vi "Main.vi"() -> ()   [LabVIEW 2015]
doc: "This template is for the Queued Message Handler design pattern.\n\nThe Event Handling Loop generates messages based on user interface actions.\n\nThe Message Handling Loop processes messages generated by the Event Handling Loop, or by other messages. The messages are string values, so new messages can be added easily to the Message Cases case structure in the Message Handling Loop. Each message cluster can also provide an optional value for Message Data, which is a variant that can be converted to whatever message-specific data is required."
uses:
  controls/UI Data.ctl
  support/Message Queue/Message Queue.lvlib
  <vilib>/Utility/error.llb/Error Cluster From Error Code.vi
  support/User Event - Stop/User Event - Stop.lvlib
  support/Message Queue/Enqueue Message (Single).vi
  <vilib>/ErrorRing/Error Ring.xnode
  <vilib>/Utility/miscctls.llb/LVPointTypeDef.ctl
  controls/Case Status.ctl
  <vilib>/addons/database/NI_Database_API.lvlib
  <userlib>/Adding Configurations and lists/Get and Set Data.lvlib
  <userlib>/origin_lib_main/DB_Interface/DB Interface.lvlib
  <userlib>/origin_lib_main/DB_Interface/DB Operations Enum.ctl
  controls/Operation type.ctl
  controls/Type.ctl
  controls/Back to Business.ctl
  controls/Declined.ctl
  controls/Program.ctl
  controls/Date to query in report.ctl
  controls/Amount in query for report.ctl
  controls/Query for report Cluster.ctl
  <vilib>/Utility/NIReport.llb/NI_report.lvclass
  <vilib>/addons/_office/NI_ReportGenerationToolkit.lvlib
  controls/Date.ctl
  controls/Add New Case.ctl
  <vilib>/addons/_office/excel.llb/Excel Easy Table (str).vi
  <vilib>/Utility/config.llb/NI_LVConfig.lvlib
  controls/Global.vi
  <vilib>/Utility/config.llb/Write Key (Path).vi
  <vilib>/Utility/config.llb/Read Key (Path).vi
  <vilib>/addons/database/Connection.llb/DB Tools Open Connec (String).vi
  <userlib>/_OpenG.lib/array/array.llb/Remove Duplicates from 1D Array (String)__ogtk.vi
  controls/Update Case.ctl
panel:
  out "error out 11":errorcluster
  out "error out 10":errorcluster
  out "Array 3":string[][](array[string])
  out "Array 2":string[][](array[string])
  out "error out 9":errorcluster
  out "Array":string[][](array[string])
  out "error out 8":errorcluster
  out "error out 7":errorcluster
  out "error out 6":errorcluster
  in  "TAT RISK":bool
  out "data Out 2":variant[][](array[variant])
  out "data 2":string[][](array[string])
  out "DB Cols Names 2":string[](array[string])
  out "error out 5":errorcluster
  out "error out":errorcluster
  out "DB Cols Names":string[](array[string])
  out "data":string[][](array[string])
  out "data Out":variant[][](array[variant])
  out "error out 4":errorcluster
  out "String":string
  out "error out 3":errorcluster
  out "error out 2":errorcluster
  in  "Exit":bool
  in  "Home Button":bool
  out "Display <Replace Me>":string
  in  "Tab Control":T1(tab)
  in  "Add New Case":bool
  in  "Existing Case":bool
  in  "Report":bool
  in  "Save Button":bool
  in  "Attachement":path
  in  "New Case":T2 {"Business Replay date" format="%<%d/%m/%Y>T"; "Next Review date" format="%<%d/%m/%Y>T"; "Stamped date" format="%<%d/%m/%Y>T"; "CAD submission date" format="%<%d/%m/%Y>T"; "decline date" format="%<%d/%m/%Y>T"; "CAM date" format="%<%d/%m/%Y>T"; "Pending risk visit date" format="%<%d/%m/%Y>T"; "Back to business 3" format="%<%d/%m/%Y>T"; "Back to business 2" format="%<%d/%m/%Y>T"; "Back to business 1" format="%<%d/%m/%Y>T"; "3rd login Date" format="%<%d/%m/%Y>T"; "2nd login Date" format="%<%d/%m/%Y>T"; "1st Login Date" format="%<%d/%m/%Y>T"}
  in  "Delete Case":bool
  in  "Query by serial":bool
  in  "Case Serial":string
  in  "Query by customer name":bool
  in  "Customer Name":string(combo)
  in  "Customer Number":string
  in  "Query by customer number":bool
  in  "Update existing Case":T9={"Customer Number"="", "UW"="", "UWTH"="", "Customer Name"="", "Program"="", "Amount"="", "CCRM"="", "CCRTH"="", "Type"="", "Case status"="Under Review", "1st Login Date"=timestamp(0 s since 1904-01-01), "2nd login Date"=timestamp(0 s since 1904-01-01), "3rd login Date"=timestamp(0 s since 1904-01-01), "Back to business 1"=timestamp(0 s since 1904-01-01), "Back to business 2"=timestamp(0 s since 1904-01-01), "Back to business 3"=timestamp(0 s since 1904-01-01), "Pending risk visit date"=timestamp(0 s since 1904-01-01), "CAM date"=timestamp(0 s since 1904-01-01), "decline date"=timestamp(0 s since 1904-01-01), "CAD submission date"=timestamp(0 s since 1904-01-01), "Stamped date"=timestamp(0 s since 1904-01-01), "Next Review date"=timestamp(0 s since 1904-01-01), "Business Replay date"=timestamp(0 s since 1904-01-01), "Comment"="", "Declined"="", "Back to business"="", "serial"=""} {"Business Replay date" format="%<%d/%m/%Y>T"; "Next Review date" format="%<%d/%m/%Y>T"; "Stamped date" format="%<%d/%m/%Y>T"; "CAD submission date" format="%<%d/%m/%Y>T"; "decline date" format="%<%d/%m/%Y>T"; "CAM date" format="%<%d/%m/%Y>T"; "Pending risk visit date" format="%<%d/%m/%Y>T"; "Back to business 3" format="%<%d/%m/%Y>T"; "Back to business 2" format="%<%d/%m/%Y>T"; "Back to business 1" format="%<%d/%m/%Y>T"; "3rd login Date" format="%<%d/%m/%Y>T"; "2nd login Date" format="%<%d/%m/%Y>T"; "1st Login Date" format="%<%d/%m/%Y>T"}
  in  "attachement":string
  in  "Open attachement":bool
  out "Case Serial 2":string
  in  "Update":bool
  in  "Reset Button":bool
  in  "Report Tab":T10(tab)
  in  "Generic Report Tab":bool
  in  "Daily Report Tab":bool
  in  "review date before 90 days":bool
  in  "Reset Button 2":bool
  in  "Report Button":bool
  in  "Back":bool
  in  "Report Cluster":T11 {"Business Replay date"."From :" format="%<%d/%m/%y>T"; "Business Replay date"."To :" format="%<%d/%m/%y>T"; "Next Review date"."From :" format="%<%d/%m/%y>T"; "Next Review date"."To :" format="%<%d/%m/%y>T"; "Stamped date"."From :" format="%<%d/%m/%y>T"; "Stamped date"."To :" format="%<%d/%m/%y>T"; "CAD submission date"."From :" format="%<%d/%m/%y>T"; "CAD submission date"."To :" format="%<%d/%m/%y>T"; "decline date"."From :" format="%<%d/%m/%y>T"; "decline date"."To :" format="%<%d/%m/%y>T"; "CAM date"."From :" format="%<%d/%m/%y>T"; "CAM date"."To :" format="%<%d/%m/%y>T"; "Pending risk visit date"."From :" format="%<%d/%m/%y>T"; "Pending risk visit date"."To :" format="%<%d/%m/%y>T"; "Back to business 3"."From :" format="%<%d/%m/%y>T"; "Back to business 3"."To :" format="%<%d/%m/%y>T"; "Back to business 2"."From :" format="%<%d/%m/%y>T"; "Back to business 2"."To :" format="%<%d/%m/%y>T"; "Back to business 1"."From :" format="%<%d/%m/%y>T"; "Back to business 1"."To :" format="%<%d/%m/%y>T"; "3rd login Date"."From :" format="%<%d/%m/%y>T"; "3rd login Date"."To :" format="%<%d/%m/%y>T"; "2nd login Date"."From :" format="%<%d/%m/%y>T"; "2nd login Date"."To :" format="%<%d/%m/%y>T"; "1st Login Date"."From :" format="%<%d/%m/%y>T"; "1st Login Date"."To :" format="%<%d/%m/%y>T"}
  in  "Back":bool
  in  "Approved Date":T12 {"From :" format="%<%d/%m/%y>T"; "To :" format="%<%d/%m/%y>T"}
  in  "Report Button 3":bool
  in  "decline date":T12 {"From :" format="%<%d/%m/%y>T"; "To :" format="%<%d/%m/%y>T"}
  # "Underwriting Pipline Submission"
  # "Attachment:"
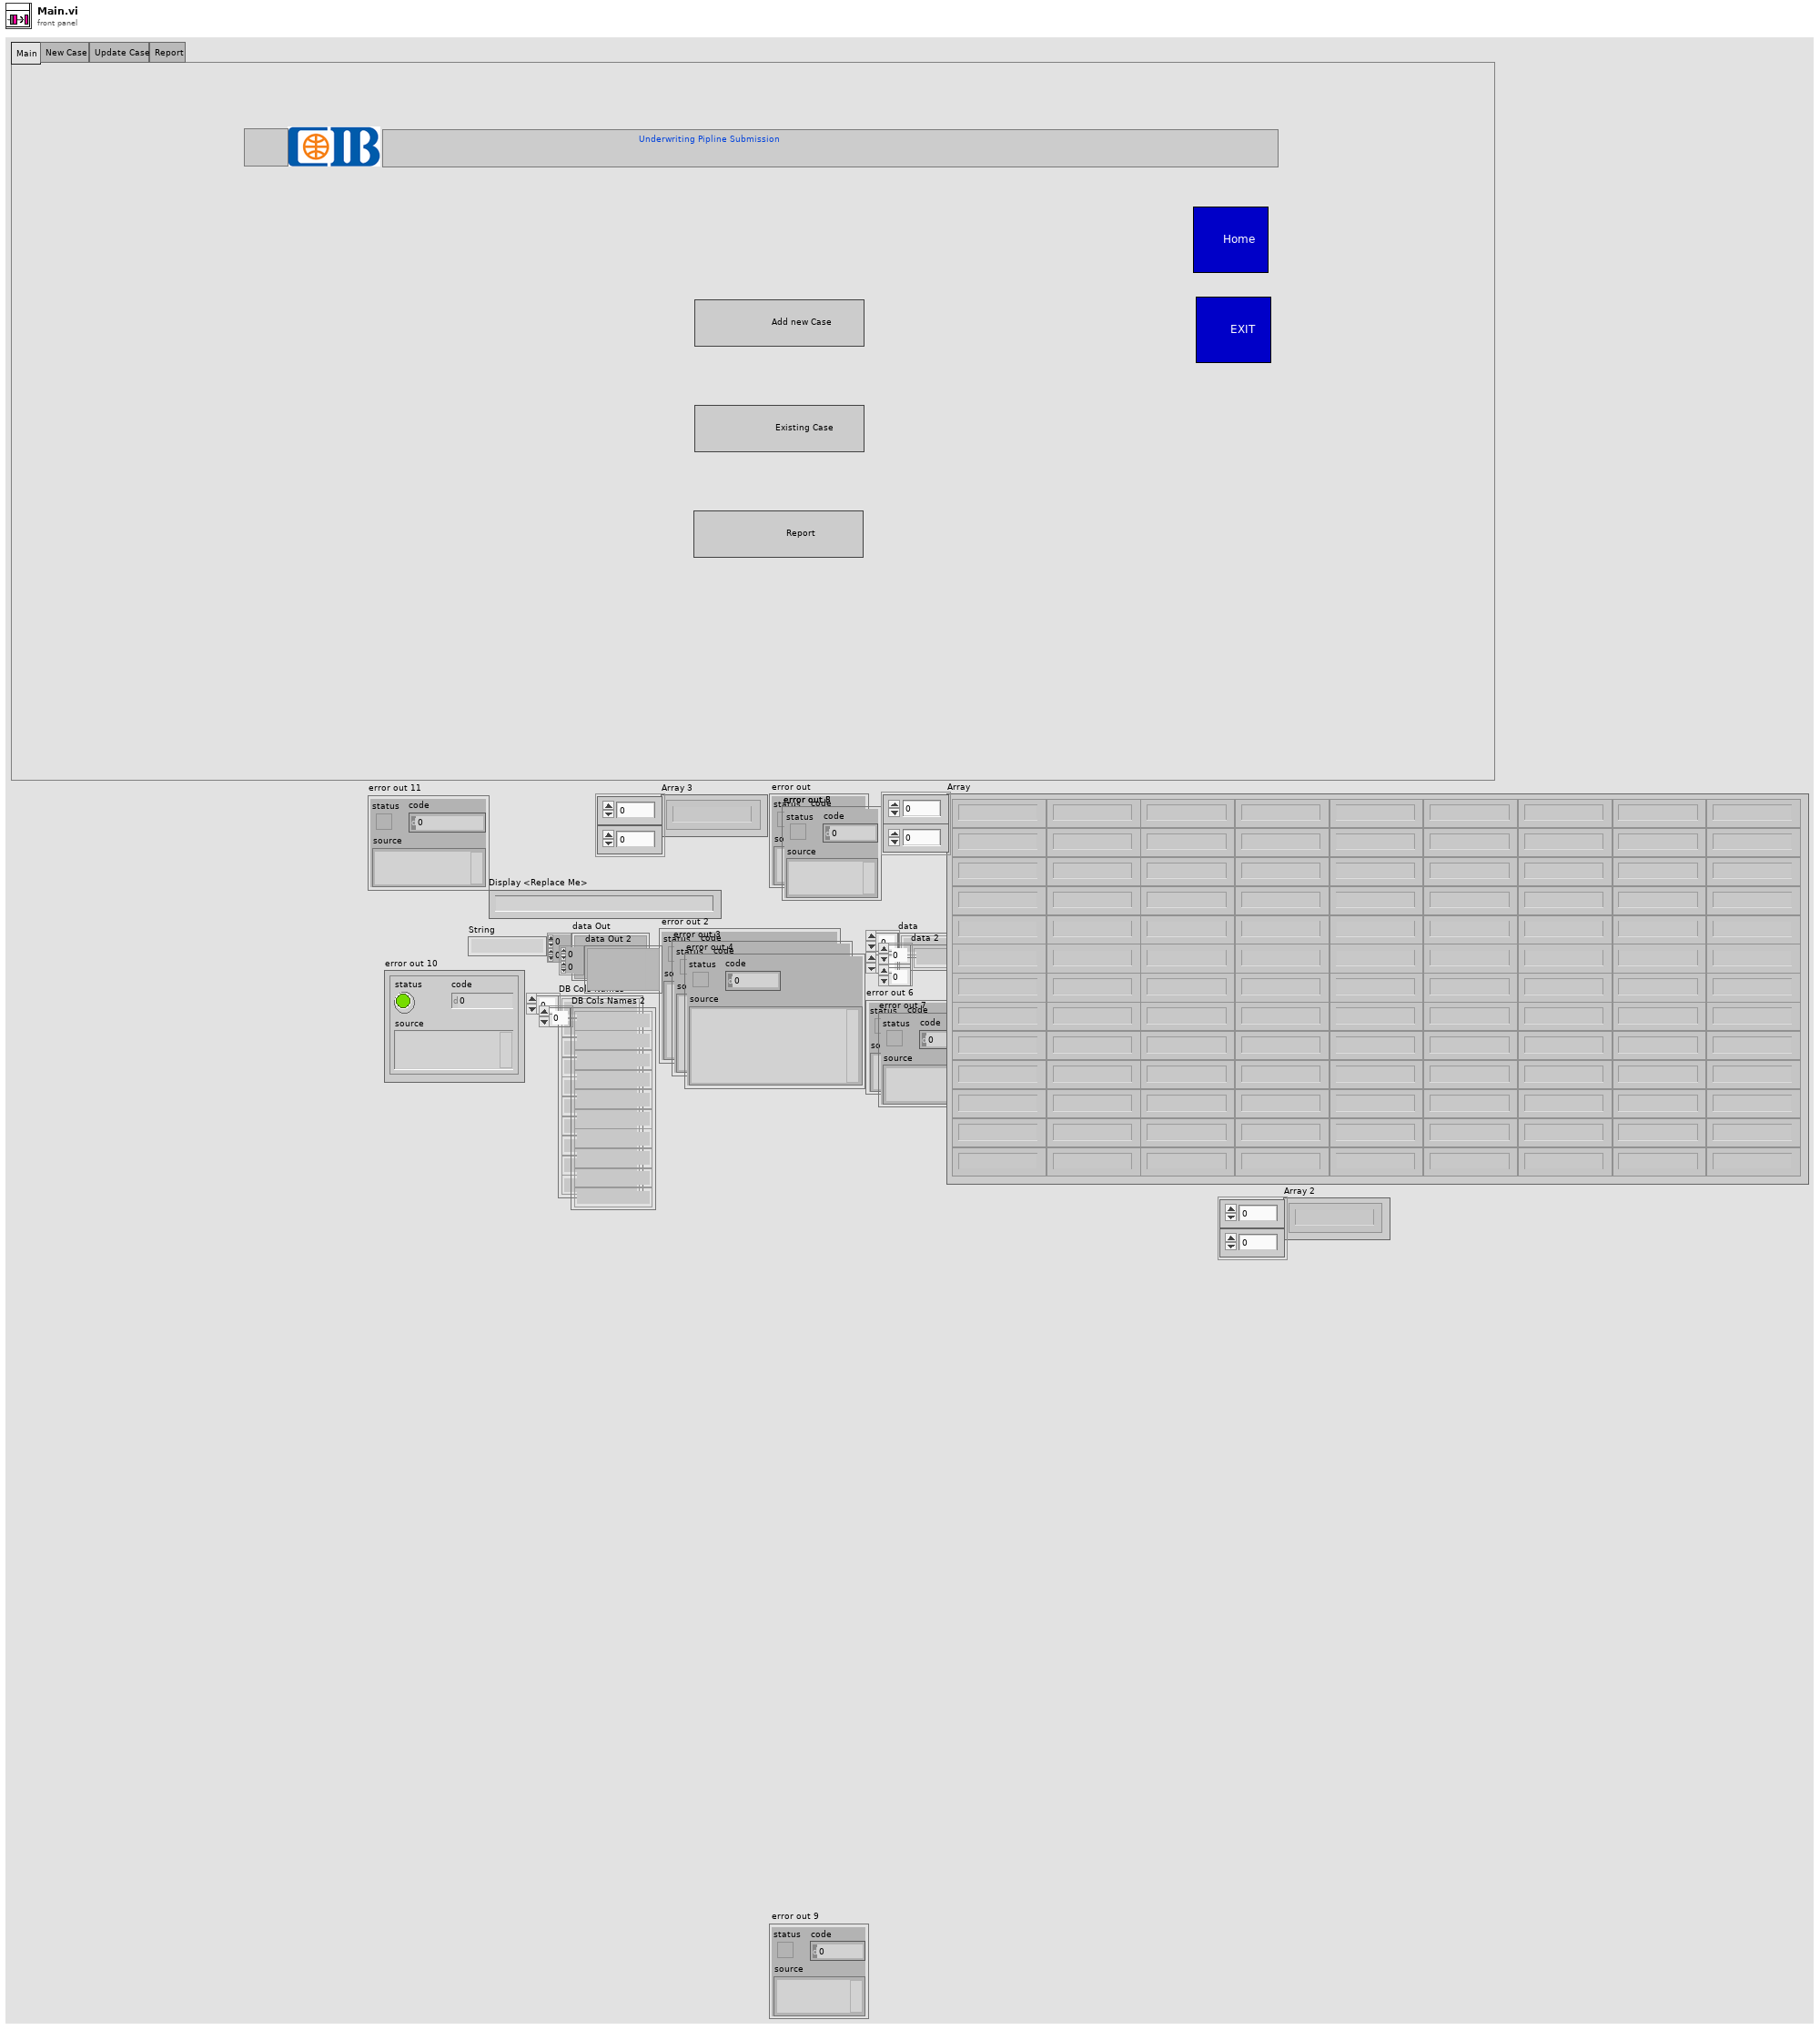
[diagram p1: front panel]
types:
  T1 = enum32{"Main", "New Case", "Update Case", "Report"}
  T2 = typedef "Add New Case.ctl" = cluster{"Customer Number":string, "UW":string, "UWTH":string, "Customer Name":string, "Program":T3, "Amount":string, "CCRM":string, "CCRTH":string, "Type":T4, "Case status":T5, "1st Login Date":T6, "2nd login Date":T6, "3rd login Date":T6, "Back to business 1":T6, "Back to business 2":T6, "Back to business 3":T6, "Pending risk visit date":T6, "CAM date":T6, "decline date":T6, "CAD submission date":T6, "Comment":string, "Stamped date":T6, "Next Review date":T6, "Declined":T7, "Back to business":T8, "serial":string, "Business Replay date":T6}
  T3 = typedef "Program.ctl" = string
  T4 = typedef "Type.ctl" = string
  T5 = typedef "Case Status.ctl" = string
  T6 = typedef "Date.ctl" = timestamp
  T7 = typedef "Declined.ctl" = string
  T8 = typedef "Back to Business.ctl" = string
  T9 = typedef "Update Case.ctl" = cluster{"Customer Number":string, "UW":string, "UWTH":string, "Customer Name":string, "Program":T3, "Amount":string, "CCRM":string, "CCRTH":string, "Type":T4, "Case status":T5, "1st Login Date":T6, "2nd login Date":T6, "3rd login Date":T6, "Back to business 1":T6, "Back to business 2":T6, "Back to business 3":T6, "Pending risk visit date":T6, "CAM date":T6, "decline date":T6, "CAD submission date":T6, "Stamped date":T6, "Next Review date":T6, "Business Replay date":T6, "Comment":string, "Declined":T7, "Back to business":T8, "serial":string}
  T10 = enum32{"Main Report", "Report 1", "Daily Report"}
  T11 = typedef "Query for report Cluster.ctl" = cluster{"UW":string, "UWTH":string, "CCRM":string, "CCRTH":string, "Type":T4, "Back to business":T8, "Declined":T7, "Program":T3, "Case status":T5, "1st Login Date":T12, "2nd login Date":T12, "3rd login Date":T12, "Business Replay date":T12, "Back to business 1":T12, "Back to business 2":T12, "Back to business 3":T12, "Next Review date":T12, "CAD submission date":T12, "CAM date":T12, "Pending risk visit date":T12, "decline date":T12, "Stamped date":T12, "Amount":T13, "Customer Number":string, "Customer Name":string, "Comment":string, "serial":string}
  T12 = typedef "Date to query in report.ctl" = cluster{"To :":timestamp, "From : ":timestamp}
  T13 = typedef "Amount in query for report.ctl" = cluster{"Amount":string, "Comparison":string}
  T14 = typedef "UI Data.ctl" = cluster{"Boolean <Replace Me>":bool, "String <Replace Me>":string, "Numeric <Replace Me>":dbl, "Do Something Ref":refnum<vi>, "Do Something Else Ref":refnum<vi>, "Data Display Ref":refnum<vi>, "Exit Button Ref":refnum<vi>}
  T15 = typedef "Message Queue.lvlib/All Message Queues.ctl" = cluster{"UI":refnum<queue>}
  T16 = typedef "LVDateTimeRec.ctl" = cluster{"fractional second":dbl, "second":i32, "minute":i32, "hour":i32, "day of month":i32, "month":i32, "year":i32, "day of week":i32, "day of year":i32, "DST":i32}
  T17 = enum8{"Enabled", "Disabled", "Disabled and Grayed Out"}
  T18 = typedef "LVPointTypeDef.ctl" = cluster{"Horizontal":i16, "Vertical":i16}
  T19 = typedef "Operation type.ctl" = enum16{"Add", "Query", "Update"}
  T20 = typedef "DB Interface.lvlib/DB Operations Enum.ctl" = enum16{"Select", "Update", "Insert", "Delete", "Fetch SQL Query", "Execute SQL Query", "Drop Table", "List Tables"}
  T21 = enum16{"Standard Report", "HTML", "Word", "Excel"}
  T22 = enum16{"maximized", "minimized", "normal", "no change"}
  T23 = typedef "NI_LVConfig.lvlib/Config Data RefNum.ctl" = refnum<k1>
  T24 = typedef "NI_Database_API.lvlib/Conn ObjectReference.ctl" = refnum<k1>
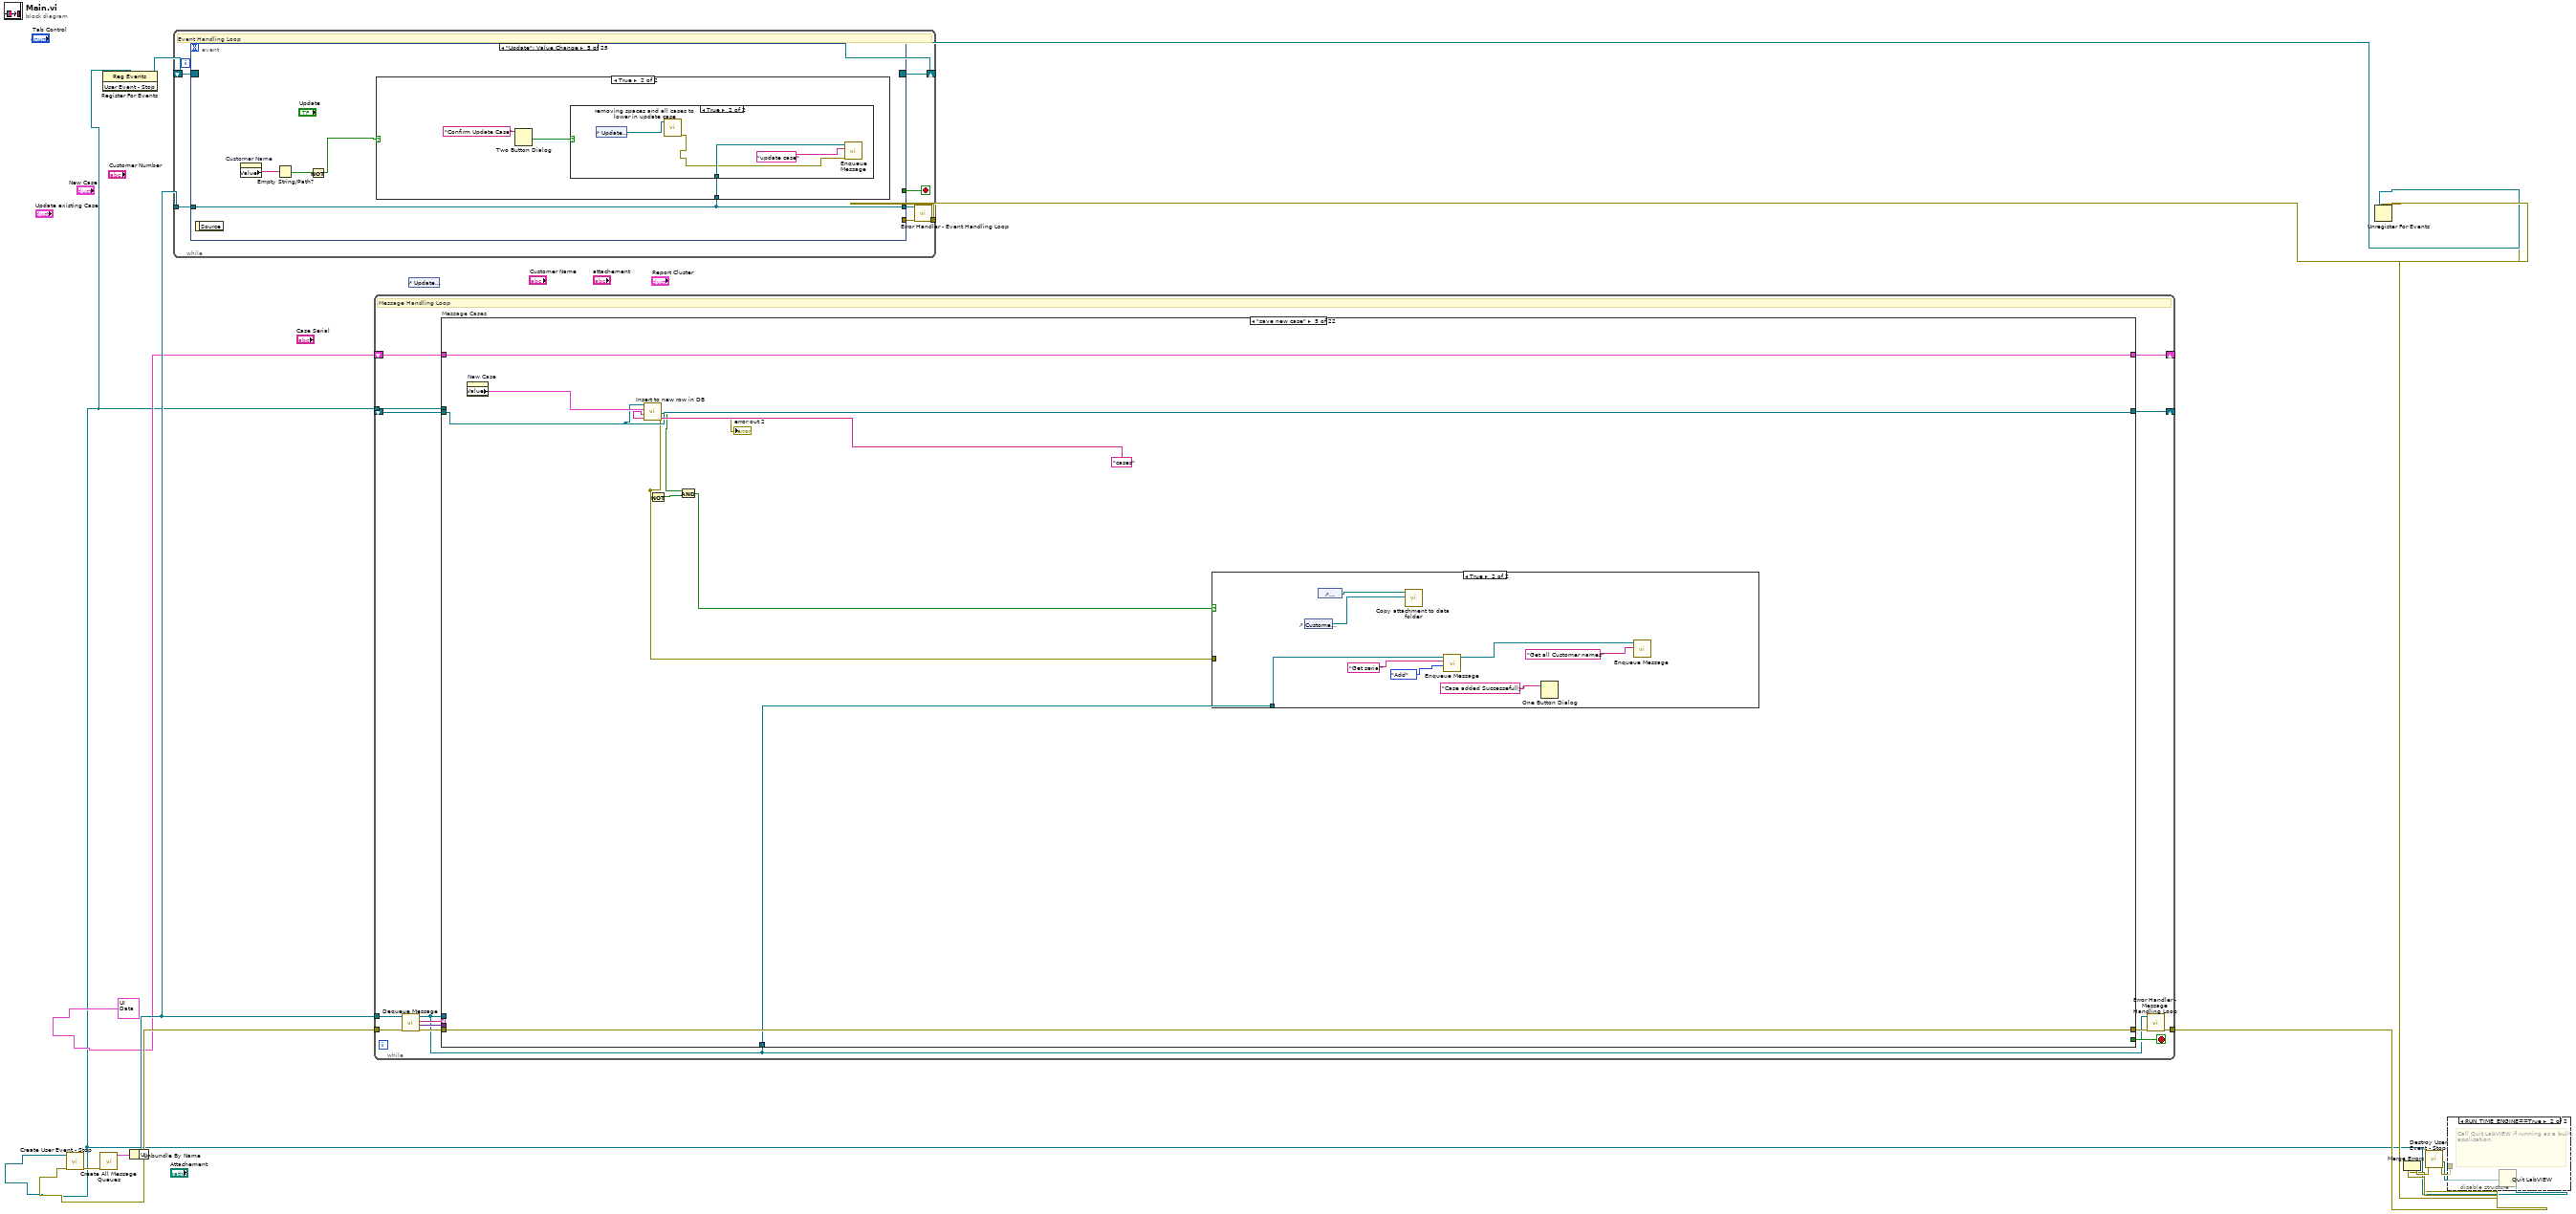
[diagram p0: block diagram]
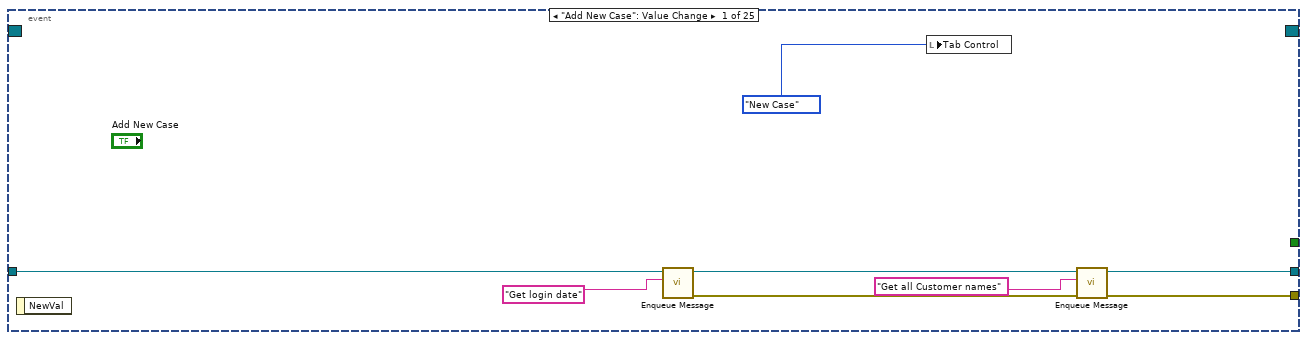
[diagram p3: hidden frame]
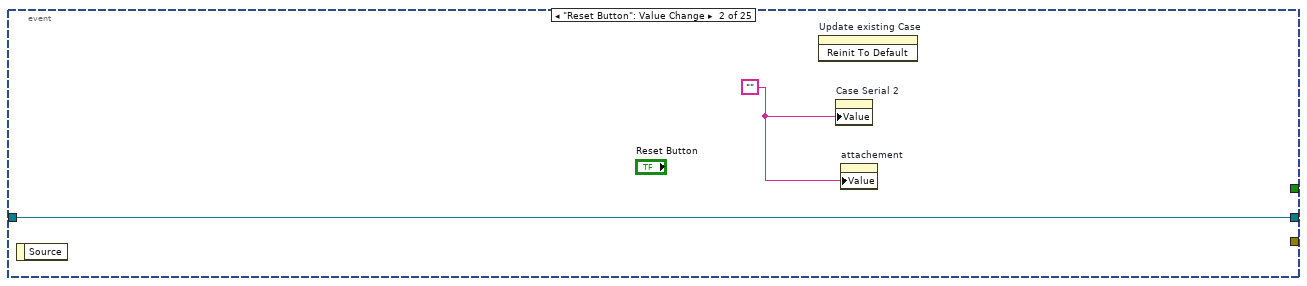
[diagram p4: hidden frame]
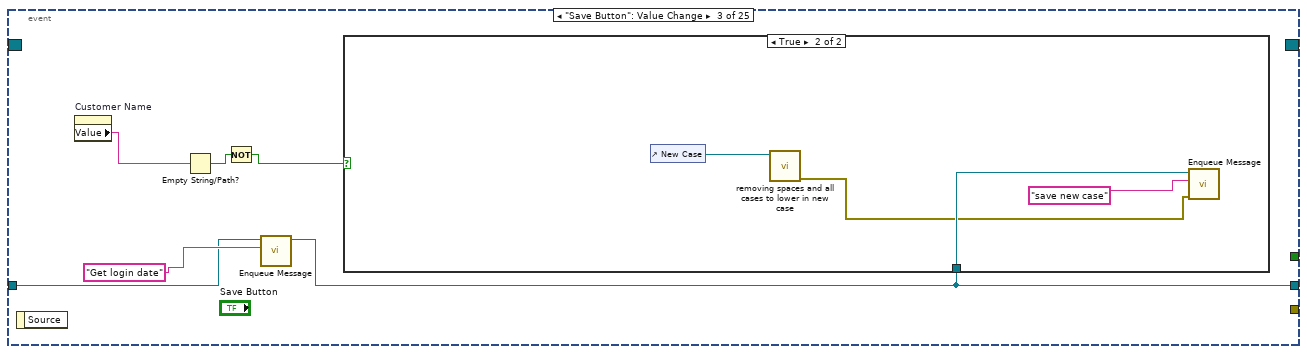
[diagram p5: hidden frame]
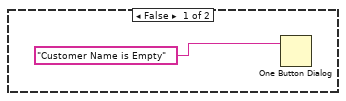
[diagram p6: hidden frame]
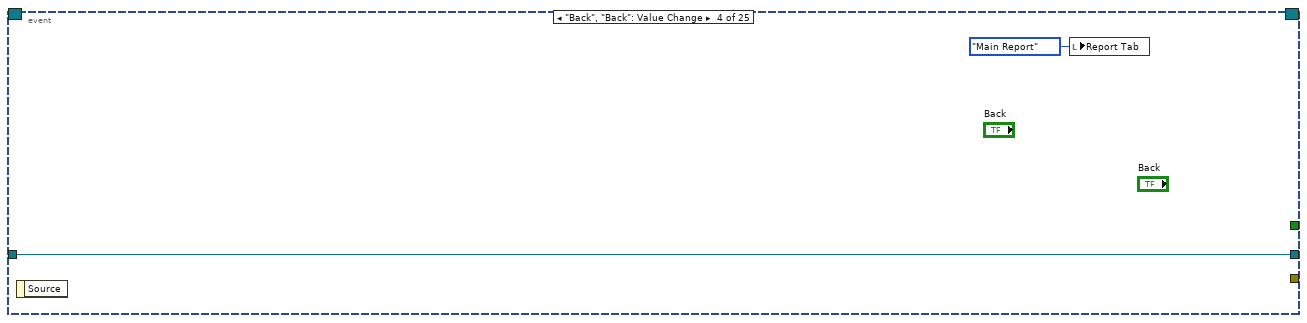
[diagram p7: hidden frame]
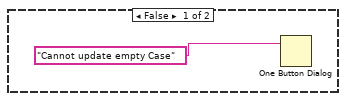
[diagram p8: hidden frame]
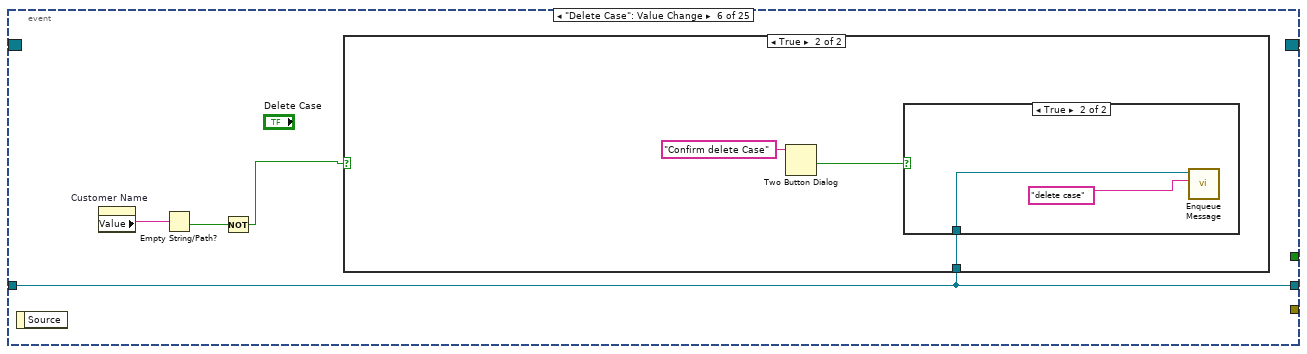
[diagram p10: hidden frame]
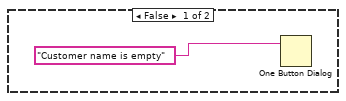
[diagram p11: hidden frame]
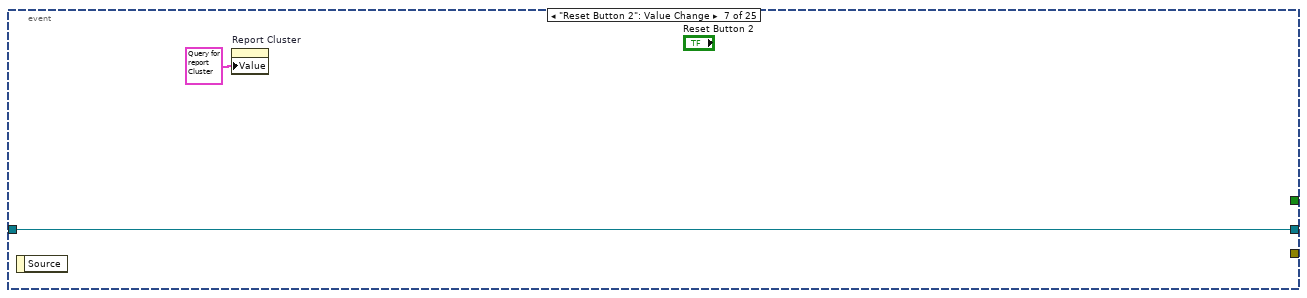
[diagram p13: hidden frame]
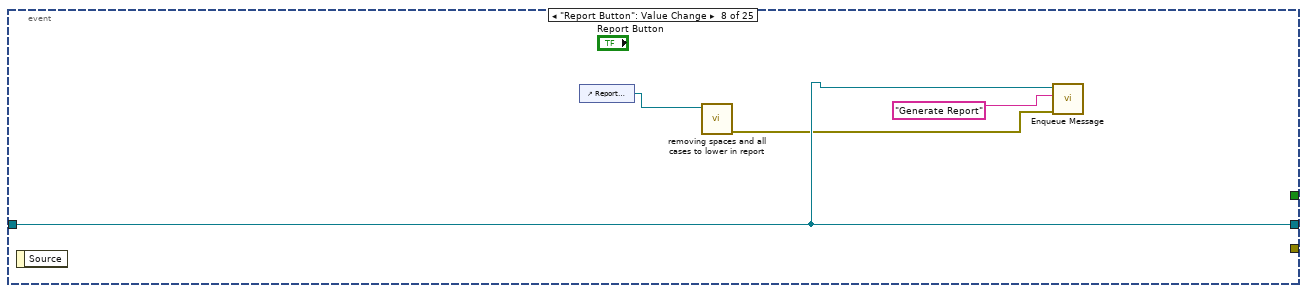
[diagram p14: hidden frame]
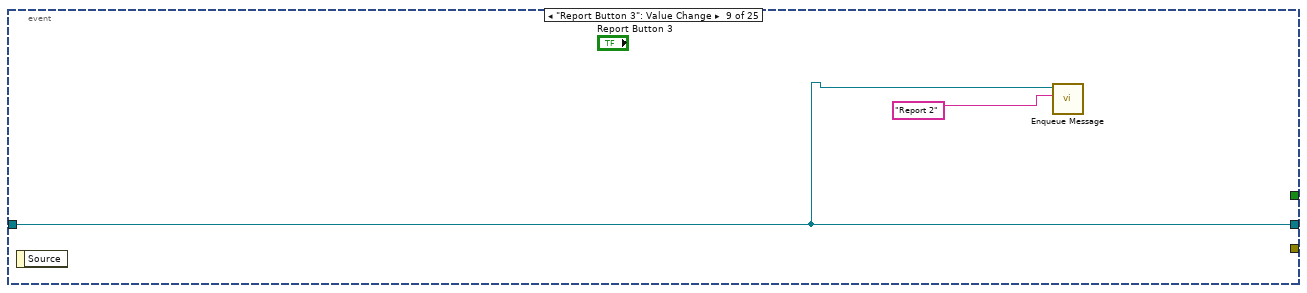
[diagram p15: hidden frame]
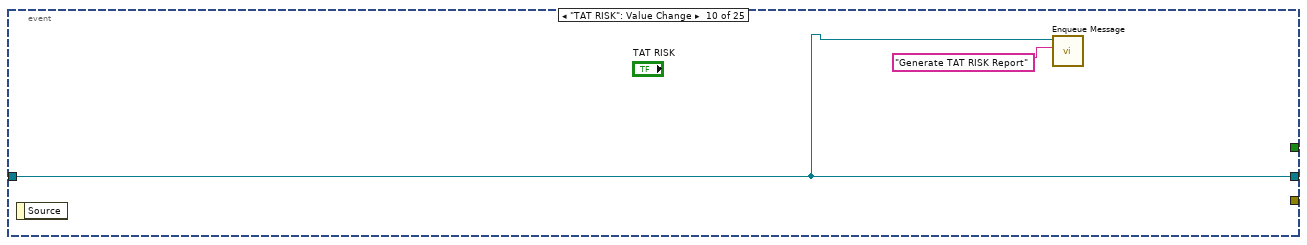
[diagram p16: hidden frame]
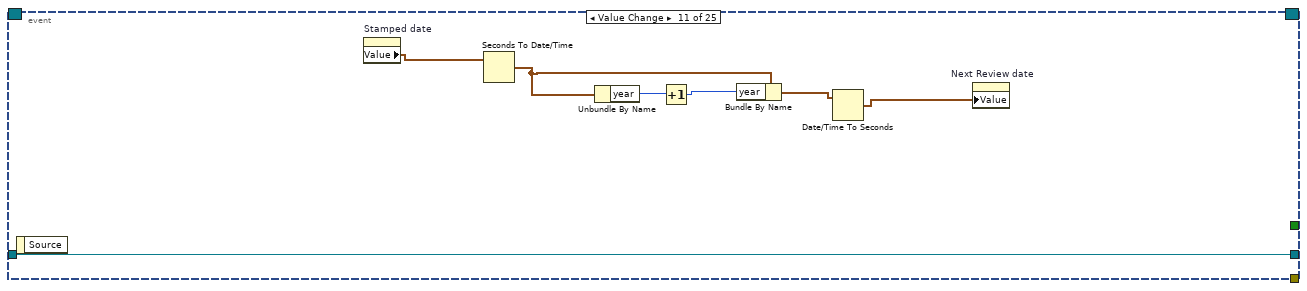
[diagram p17: hidden frame]
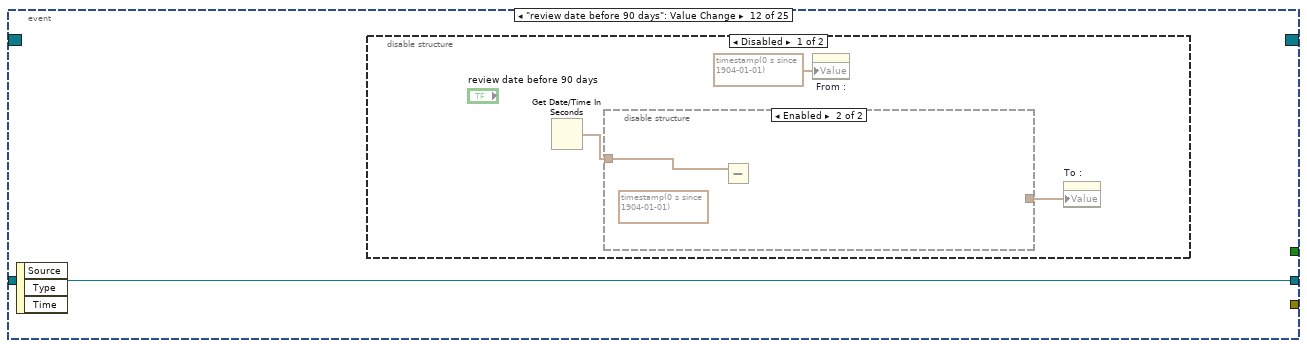
[diagram p18: hidden frame]
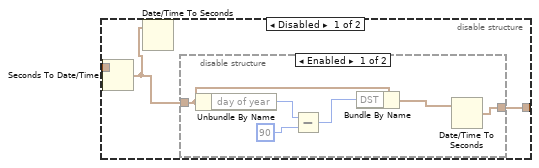
[diagram p19: hidden frame]
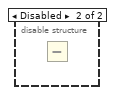
[diagram p20: hidden frame]
diagram:
  n1 = call "Create User Event - Stop.vi"() -> ("error out"=w9:errorcluster, "User Event - Stop"=w1:refnum<user-event>)  [unwired: 10 in]
  n2 = call "Create All Message Queues.vi"("error in (no error)"=w9) -> ("error out"=w13:errorcluster, "Message Queues out"=w12:T15)  [unwired: 9 in]
  n3 = register-events(w1) -> (reference out=w2:refnum<event-registration>)  [unwired: 2 in, 1 out]
  n4 = Unbundle By Name(w12) -> ("UI"=w10:refnum<queue>)
  n5 = while {
    tunnel: w10 -> [w20]
    shift-right: [w18] -> w6
    shift-left: w2 -> [w19]
    tunnel: [w14] -> w3
    stop <- w16 stop-if-true
    # "Event Handling Loop"
    n6 = event shown="[4] \"Update\": Value Change" {
      selector: w19 -> [_ _ _ _ _ _ _ _ _ _ _ _ _ _ _ _ _ _ _ _ _ _ _ _ _]
      dyn-events: [_ _ _ _ _ _ _ _ _ _ _ _ _ _ _ _ _ _ _ _ _ _ _ _ _] -> w18
      timeout: _ -> [_ _ _ _ _ _ _ _ _ _ _ _ _ _ _ _ _ _ _ _ _ _ _ _ _]
      tunnel: [_ _ _ _ _ _ _ _ _ _ _ _ _ _ _ _ _ _ _ _ _ _ _ _ TRUE ("Discard?")] -> w16
      tunnel: w20 -> [w28 w30 w32 w43 w47 w59 w67 w70 w72 w74 w82 w83 w111 w118 w121 w125 w132 w138 w141 w144 w146 w151 w153 w158 w161]
      tunnel: [w21 _ _ _ _ _ _ _ _ _ _ _ _ _ _ _ w129 w135 _ _ _ w150 _ w157 _] -> w17
      tunnel: [w23 w30 w31 w43 w47 w59 w67 w70 w72 w74 w82 w83 w111 w118 w121 w125 w131 w137 w141 w144 w146 w149 w153 w156 w161] -> w15
      event "Add New Case": Value Change {
        n7 = event-data() -> ()  [unwired: 1 in, 1 out]
        n8 = call-poly "Enqueue Message.vi"("Message"="Get login date", "Message Queue"=w28) -> ("error out"=w22:errorcluster, "dup Message Queue"=w24:refnum<queue>)  [unwired: 8 in]
        n9 = local write "Tab Control"(T1."New Case" ("Tab Control")) -> ()
        n10 = call-poly "Enqueue Message.vi"("error in (no error)"=w22, "Message"="Get all Customer names", "Message Queue"=w24) -> ("error out"=w21:errorcluster, "dup Message Queue"=w23:refnum<queue>)  [unwired: 7 in]
      }
      event "Reset Button": Value Change {
        w29 = ""
        n11 = event-data() -> ()  [unwired: 1 in, 1 out]
        n12 = invoke on="Update existing Case" class="Clust (strict)" method="Reinit To Default"() -> ()  [unwired: 3 in, 3 out]
        n13 = property on="Case Serial 2" class="Str"("Value"=w29) -> ()  [unwired: 2 in, 2 out]
        n14 = property on="attachement" class="Str"("Value"=w29) -> ()  [unwired: 2 in, 2 out]
      }
      event "Save Button": Value Change {
        n15 = event-data() -> ()  [unwired: 1 in, 1 out]
        n16 = property on="Customer Name" class="Str"() -> ("Value"=w36:string)  [unwired: 2 in, 2 out]
        n17 = Empty String/Path?(string/path=w36) -> (empty?=w35:bool)
        n18 = Not(x=w35) -> (.not. x?=w34:bool)
        n19 = call-poly "Enqueue Message.vi"("Message"="Get login date", "Message Queue"=w32) -> ("dup Message Queue"=w31:refnum<queue>)  [unwired: 8 in, 1 out]
        n20 = case shown="True" w34 {
          tunnel: w31 -> [_ w40]
          frame False {
            n21 = One Button Dialog(message="Customer Name is Empty") -> ()  [unwired: 1 in, 1 out]
          }
          frame True {
            n22 = control-ref of="New Case"() -> (w39:refnum<vi>)
            n23 = call "removing spaces and all cases to lower in new case.vi"("New Case"=w39) -> ("Error Out"=w38:errorcluster)  [unwired: 10 in]
            n24 = call-poly "Enqueue Message.vi"("error in (no error)"=w38, "Message"="save new case", "Message Queue"=w40) -> ()  [unwired: 7 in, 2 out]
          }
        }
      }
      event "Back", "Back": Value Change {
        n25 = event-data() -> ()  [unwired: 1 in, 1 out]
        n26 = local write "Report Tab"(T10."Main Report" ("Report Tab")) -> ()
      }
      event "Update": Value Change {
        n27 = event-data() -> ()  [unwired: 1 in, 1 out]
        n28 = property on="Customer Name" class="Str"() -> ("Value"=w46:string)  [unwired: 2 in, 2 out]
        n29 = Empty String/Path?(string/path=w46) -> (empty?=w45:bool)
        n30 = Not(x=w45) -> (.not. x?=w44:bool)
        n31 = case shown="True" w44 {
          tunnel: w47 -> [_ w51]
          frame False {
            n32 = One Button Dialog(message="Cannot update empty Case") -> ()  [unwired: 1 in, 1 out]
          }
          frame True {
            n33 = Two Button Dialog(message="Confirm Update Case") -> (T button?=w50:bool)  [unwired: 2 in]
            n34 = case shown="True" w50 {
              tunnel: w51 -> [_ w54]
              frame False {
              }
              frame True {
                n35 = control-ref of="Update existing Case"() -> (w53:refnum<vi>)
                n36 = call "removing spaces and all cases to lower in update case.vi"("Update existing Case"=w53) -> ("Error Out"=w52:errorcluster)  [unwired: 10 in]
                n37 = call-poly "Enqueue Message.vi"("error in (no error)"=w52, "Message"="update case", "Message Queue"=w54) -> ()  [unwired: 7 in, 2 out]
              }
            }
          }
        }
      }
      event "Delete Case": Value Change {
        n38 = event-data() -> ()  [unwired: 1 in, 1 out]
        n39 = property on="Customer Name" class="Str"() -> ("Value"=w58:string)  [unwired: 2 in, 2 out]
        n40 = Empty String/Path?(string/path=w58) -> (empty?=w57:bool)
        n41 = Not(x=w57) -> (.not. x?=w56:bool)
        n42 = case shown="True" w56 {
          tunnel: w59 -> [_ w63]
          frame False {
            n43 = One Button Dialog(message="Customer name is empty") -> ()  [unwired: 1 in, 1 out]
          }
          frame True {
            n44 = Two Button Dialog(message="Confirm delete Case") -> (T button?=w62:bool)  [unwired: 2 in]
            n45 = case shown="True" w62 {
              tunnel: w63 -> [_ w64]
              frame False {
              }
              frame True {
                n46 = call-poly "Enqueue Message.vi"("Message"="delete case", "Message Queue"=w64) -> ()  [unwired: 8 in, 2 out]
              }
            }
          }
        }
      }
      event "Reset Button 2": Value Change {
        n47 = event-data() -> ()  [unwired: 1 in, 1 out]
        n48 = property on="Report Cluster" class="Clust (strict)"("Value"=T11 {"UW"="", "UWTH"="", "CCRM"="", "CCRTH"="", "Type"="", "Back to business"="", "Declined"="", "Program"="", "Case status"="", "1st Login Date"={"To :"=timestamp(0 s since 1904-01-01), "From : "=timestamp(0 s since 1904-01-01)}, "2nd login Date"={"To :"=timestamp(0 s since 1904-01-01), "From : "=timestamp(0 s since 1904-01-01)}, "3rd login Date"={"To :"=timestamp(0 s since 1904-01-01), "From : "=timestamp(0 s since 1904-01-01)}, "Business Replay date"={"To :"=timestamp(0 s since 1904-01-01), "From : "=timestamp(0 s since 1904-01-01)}, "Back to business 1"={"To :"=timestamp(0 s since 1904-01-01), "From : "=timestamp(0 s since 1904-01-01)}, "Back to business 2"={"To :"=timestamp(0 s since 1904-01-01), "From : "=timestamp(0 s since 1904-01-01)}, "Back to business 3"={"To :"=timestamp(0 s since 1904-01-01), "From : "=timestamp(0 s since 1904-01-01)}, "Next Review date"={"To :"=timestamp(0 s since 1904-01-01), "From : "=timestamp(0 s since 1904-01-01)}, "CAD submission date"={"To :"=timestamp(0 s since 1904-01-01), "From : "=timestamp(0 s since 1904-01-01)}, "CAM date"={"To :"=timestamp(0 s since 1904-01-01), "From : "=timestamp(0 s since 1904-01-01)}, "Pending risk visit date"={"To :"=timestamp(0 s since 1904-01-01), "From : "=timestamp(0 s since 1904-01-01)}, "decline date"={"To :"=timestamp(0 s since 1904-01-01), "From : "=timestamp(0 s since 1904-01-01)}, "Stamped date"={"To :"=timestamp(0 s since 1904-01-01), "From : "=timestamp(0 s since 1904-01-01)}, "Amount"={"Amount"="", "Comparison"=""}, "Customer Number"="", "Customer Name"="", "Comment"="", "serial"=""} ("Update existing Case 2")) -> ()  [unwired: 2 in, 2 out]
      }
      event "Report Button": Value Change {
        n49 = event-data() -> ()  [unwired: 1 in, 1 out]
        n50 = control-ref of="Report Cluster"() -> (w69:refnum<vi>)
        n51 = call "removing spaces and all cases to lower in report.vi"("Report Cluster"=w69) -> ("Error Out"=w68:errorcluster)  [unwired: 10 in]
        n52 = call-poly "Enqueue Message.vi"("error in (no error)"=w68, "Message"="Generate Report", "Message Queue"=w70) -> ()  [unwired: 7 in, 2 out]
      }
      event "Report Button 3": Value Change {
        n53 = event-data() -> ()  [unwired: 1 in, 1 out]
        n54 = call-poly "Enqueue Message.vi"("Message"="Report 2", "Message Queue"=w72) -> ()  [unwired: 8 in, 2 out]
      }
      event "TAT RISK": Value Change {
        n55 = event-data() -> ()  [unwired: 1 in, 1 out]
        n56 = call-poly "Enqueue Message.vi"("Message"="Generate TAT RISK Report", "Message Queue"=w74) -> ()  [unwired: 8 in, 2 out]
      }
      event Value Change {
        n57 = event-data() -> ()  [unwired: 1 in, 1 out]
        n58 = property on="Stamped date" class="AbsTime (strict)"() -> ("Value"=w76:T6)  [unwired: 2 in, 2 out]
        n59 = Seconds To Date/Time(time stamp (now)=w76) -> (date time rec=w80:T16)  [unwired: 1 in]
        n60 = Unbundle By Name(w80) -> ("year"=w81:i32)
        n61 = Increment(x=w81) -> (x+1=w79:i32)
        n62 = Bundle By Name(cluster=w80, "year"=w79) -> (w78:T16)
        n63 = Date/Time To Seconds(2:w78) -> (0:w77:timestamp)  [unwired: 1 in]
        n64 = property on="Next Review date" class="AbsTime (strict)"("Value"=w77) -> ()  [unwired: 2 in, 2 out]
      }
      event "review date before 90 days": Value Change {
        n65 = event-data() -> ()  [unwired: 1 in, 3 out]
        n66 = disable-structure shown="Disabled" {
          frame Disabled {
            n67 = Get Date/Time In Seconds() -> (seconds since 1Jan1904=w85:timestamp)
            n68 = disable-structure shown="Enabled" {
              disable-tunnel: w85 -> [w89 w96]
              disable-tunnel: [w88 _] -> w84
              frame Disabled {
                n69 = Seconds To Date/Time(time stamp (now)=w89) -> (date time rec=w87:T16)  [unwired: 1 in]
                n70 = Date/Time To Seconds(2:w87) -> ()  [unwired: 1 in, 1 out]
                n71 = disable-structure shown="Enabled" {
                  disable-tunnel: w87 -> [w95 _]
                  disable-tunnel: [w90 _] -> w88
                  frame Enabled {
                    n72 = Unbundle By Name(w95) -> ("day of year"=w94:i32)
                    n73 = Subtract(x=w94, y=90) -> (x-y=w92:i32)
                    n74 = Bundle By Name(cluster=w95, "DST"=w92) -> (w91:T16)
                    n75 = Date/Time To Seconds(2:w91) -> (0:w90:timestamp)  [unwired: 1 in]
                  }
                  frame Disabled {
                    n76 = Subtract() -> ()  [unwired: 2 in, 1 out]
                  }
                }
              }
              frame Enabled {
                (unwired) timestamp(0 s since 1904-01-01) ("seconds since 1Jan1904")
                n77 = Subtract(x=w96) -> ()  [unwired: 1 in, 1 out]
              }
            }
            n78 = property on="From :" class="AbsTime (strict)"("Value"=timestamp(0 s since 1904-01-01)) -> ()  [unwired: 2 in, 2 out]
            n79 = property on="To :" class="AbsTime (strict)"("Value"=w84) -> ()  [unwired: 2 in, 2 out]
          }
          frame Enabled {
          }
        }
      }
      event "Open attachement": Value Change {
        n80 = event-data() -> ()  [unwired: 1 in, 1 out]
        n81 = global read "Global.vi" "attachment path"() -> (w97:path)
        n82 = property on="attachement" class="Str"() -> ("Value"=w102:string)  [unwired: 2 in, 2 out]
        n83 = call <vilib>:"Is Path and Not Empty.vi"("path"=w97) -> ("Is Path and Not Empty?"=w98:bool)  [unwired: 4 in]
        n84 = property on="Customer Name" class="Str"() -> ("Value"=w100:string)  [unwired: 2 in, 2 out]
        n85 = case shown="True" w98 {
          tunnel: [w114 w115] -> w99
          tunnel: w97 -> [_ w115]
          frame False {
            n86 = call <vilib>:"Application Directory.vi"() -> ("Application Directory"=w113:path)
            n87 = Build Path(base path=w113, name or relative path="data\\attachment\\") -> (appended path=w114:path)
          }
          frame True {
          }
        }
        n88 = Concatenate Strings(w100, "\\", w102) -> (w110:string)
        n89 = Build Path(base path=w99, name or relative path=w110) -> (appended path=w103:path)
        n90 = Path To String(path=w103) -> (string=w108:string)
        n91 = Concatenate Strings("cmd  /c \"", w108, "\"") -> (w106:string)
        n92 = call <vilib>:"System Exec.vi"("run minimized? (F)"=TRUE, "wait until completion? (T)"=FALSE, "command line"=w106) -> ()  [unwired: 5 in, 4 out]
      }
      event "Query by customer number": Value Change {
        n93 = event-data() -> ()  [unwired: 1 in, 1 out]
        n94 = property on="Customer Number" class="Str"() -> ("Value"=w117:string)  [unwired: 2 in, 2 out]
        n95 = Empty String/Path?(string/path=w117) -> (empty?=w116:bool)
        n96 = case shown="False" w116 {
          tunnel: w118 -> [w119 _]
          frame False {
            n97 = call-poly "Enqueue Message.vi"("Message"="Query by customer number", "Message Queue"=w119) -> ()  [unwired: 8 in, 2 out]
          }
          frame True {
          }
        }
      }
      event "Query by serial": Value Change {
        n98 = event-data() -> ()  [unwired: 1 in, 1 out]
        n99 = call-poly "Enqueue Message.vi"("Message"="Query by serial", "Message Queue"=w121) -> ()  [unwired: 8 in, 2 out]
      }
      event "Query by customer name": Value Change {
        n100 = event-data() -> ()  [unwired: 1 in, 1 out]
        n101 = property on="Customer Name" class="CmbBox"() -> ("Value"=w124:string)  [unwired: 2 in, 2 out]
        n102 = Empty String/Path?(string/path=w124) -> (empty?=w123:bool)
        n103 = case shown="False" w123 {
          tunnel: w125 -> [w126 _]
          frame False {
            n104 = call-poly "Enqueue Message.vi"("Message"="Query by customer name", "Message Queue"=w126) -> ()  [unwired: 8 in, 2 out]
          }
          frame True {
          }
        }
      }
      event "Existing Case": Value Change {
        n105 = event-data() -> ()  [unwired: 1 in, 1 out]
        n106 = call-poly "Enqueue Message.vi"("Message"="Get all Customer names", "Message Queue"=w132) -> ("error out"=w129:errorcluster, "dup Message Queue"=w131:refnum<queue>)  [unwired: 8 in]
        n107 = local write "Tab Control"(T1."Update Case" ("Tab Control")) -> ()
      }
      event "Report": Value Change {
        n108 = event-data() -> ()  [unwired: 1 in, 1 out]
        n109 = call-poly "Enqueue Message.vi"("Message"="Get all Customer names", "Message Queue"=w138) -> ("error out"=w135:errorcluster, "dup Message Queue"=w137:refnum<queue>)  [unwired: 8 in]
        n110 = local write "Report Tab"(T10."Main Report" ("Report Tab")) -> ()
        n111 = local write "Tab Control"(T1."Report" ("Tab Control")) -> ()
      }
      event "Generic Report Tab": Value Change {
        n112 = event-data() -> ()  [unwired: 1 in, 1 out]
        n113 = local write "Report Tab"(T10."Report 1" ("Report Tab")) -> ()
        n114 = local write "Tab Control"(T1."Report" ("Tab Control")) -> ()
      }
      event "Daily Report Tab": Value Change {
        n115 = event-data() -> ()  [unwired: 1 in, 1 out]
        n116 = local write "Report Tab"(T10."Daily Report" ("Report Tab")) -> ()
        n117 = local write "Tab Control"(T1."Report" ("Tab Control")) -> ()
      }
      event "Home Button": Value Change {
        n118 = event-data() -> ()  [unwired: 1 in, 1 out]
        n119 = local write "Tab Control"(T1."Main" ("Tab Control")) -> ()
      }
      event Panel Close? {
        # "Send the 'Confirm Quit' message if the user closes the panel of the VI. Discard the event so the 'Confirm Quit' message has a chance to run."
        n120 = event-data() -> ()  [unwired: 1 in, 1 out]
        n121 = call-poly "Enqueue Message.vi"("Priority Message? (F)"=TRUE, "Message"="Confirm Quit", "Message Queue"=w151) -> ("error out"=w150:errorcluster, "dup Message Queue"=w149:refnum<queue>)  [unwired: 7 in]
        n122 = event-data("Discard?"=TRUE) -> ()  [unwired: 1 in, 1 out]
      }
      event Application Instance Close {
        # "#CodeRecommended - When a project closes, all VIs within that project are aborted and leave memory. However, any code placed in this event frame is guaranteed to run to completion, so add any cleanup code that absolutely must happen here."
        n123 = event-data() -> ()  [unwired: 1 in, 1 out]
      }
      event "Exit": Value Change {
        n124 = event-data() -> ()  [unwired: 1 in, 1 out]
        n125 = call-poly "Enqueue Message.vi"("Priority Message? (F)"=TRUE, "Message"="Exit", "Message Queue"=w158) -> ("error out"=w157:errorcluster, "dup Message Queue"=w156:refnum<queue>)  [unwired: 7 in]
      }
      event User Event {
        # "The Message Handling Loop processed an \"Exit\" message, which fired this event to stop the Event Handling Loop."
        n126 = event-data() -> ()  [unwired: 1 in, 1 out]
        n127 = local write "Display <Replace Me>"("\"Exit\" button pressed" ("VI Stopped")) -> ()
      }
    }
    n128 = call "Error Handler - Event Handling Loop.vi"("error in (no error)"=w17, "Message Queue"=w15) -> ("dup error in"=w14:errorcluster)  [unwired: 8 in, 1 out]
  }
  n129 = while {
    tunnel: w10 -> [w167]
    shift-right: [w174] -> _
    shift-left: T14 {"Boolean <Replace Me>"=FALSE, "String <Replace Me>"="", "Numeric <Replace Me>"=0.0, "Do Something Ref"=refnum, "Do Something Else Ref"=refnum, "Data Display Ref"=refnum, "Exit Button Ref"=refnum} ("Data Cluster") -> [w175]
    tunnel: w1 -> [w172]
    tunnel: w13 -> [w171]
    tunnel: [w166] -> w11
    shift-right: [w164] -> _
    shift-left: _ -> [w163]
    stop <- w173 stop-if-true
    # "Message Handling Loop"
    n130 = call "Dequeue Message.vi"("error in (no error)"=w171, "Message Queue"=w167) -> ("error out"=w170:errorcluster, "Message Data"=w168:variant, "Message"=w169:string, "dup Message Queue"=w162:refnum<queue>)  [unwired: 6 in]
    n131 = case "Message Cases" shown="\"save new case\"" w169 {
      selector: w169 -> [_ _ _ _ _ _ _ _ _ _ _ _ _ _ _ _ _ _ _ _ _ w646]
      tunnel: w162 -> [w184 _ _ _ _ _ _ w319 _ w351 w368 _ _ _ _ w600 _ _ w624 _ w644 _]
      tunnel: w170 -> [w191 w210 w231 w252 w272 w298 w313 w326 w344 w358 w373 w394 w406 w464 w569 w602 w610 w620 w628 w632 w637 _]
      tunnel: [w192 w210 w232 w253 w272 w298 w313 w326 w344 w358 w373 w394 w406 w464 w569 w603 w611 w614 w626 w630 w640 w647] -> w165
      tunnel: w175 -> [w190 w209 w233 w254 w271 w297 w312 w325 w343 w357 w372 w393 w405 w463 w568 w604 w612 w619 w627 w631 w643 w648]
      tunnel: [w189 w209 w233 w254 w271 w297 w312 w325 w343 w357 w372 w393 w405 w463 w568 w604 w612 w619 w627 w631 w643 w648] -> w174
      tunnel: [_ _ _ _ _ _ _ _ _ _ _ _ _ _ _ _ _ _ _ _ TRUE _] -> w173
      tunnel: w168 -> [_ _ _ w241 _ _ _ _ _ _ _ _ _ _ _ _ w609 w618 _ _ w634 _]
      tunnel: w172 -> [_ _ _ _ _ _ _ _ _ _ _ _ _ _ _ _ _ _ _ _ w639 _]
      tunnel: [w176 w207 w230 w251 w268 w295 w311 w323 w342 w355 w370 w391 w397 w441 w565 w597 w605 w613 w621 w629 w633 w645] -> w164
      tunnel: w163 -> [w176 _ w230 w251 w268 w295 w311 w323 w342 w355 w370 w391 w397 w441 w565 w597 w605 w613 w621 w629 w633 w645]
      tunnel: w162 -> [_ _ _ _ w263 _ _ _ _ _ _ _ _ _ _ _ _ _ _ _ _ _]
      frame "Initialize" {
        # "Initialize - All initialization work should take place in this message, since other loops can potentially enqueue messages that execute immediately after this one."
        n132 = control-ref of="Exit"() -> (w182:refnum<vi>)
        n133 = control-ref of="Add New Case"() -> (w188:refnum<vi>)
        n134 = control-ref of="Existing Case"() -> (w187:refnum<vi>)
        n135 = control-ref of="Display <Replace Me>"() -> (w186:refnum<vi>)
        n136 = control-ref of="Pane"() -> (w181:refnum<vi>)
        n137 = property on="Case status" class="CmbBox (strict)"("Value"=T5 "Under Review", "DisabledEnum"=T17."Disabled and Grayed Out" ("Disabled")) -> ()  [unwired: 2 in, 2 out]
        n138 = Bundle By Name(cluster=w190, "Do Something Ref"=w188, "Do Something Else Ref"=w187, "Data Display Ref"=w186, "Exit Button Ref"=w182, "String <Replace Me>"="Initial Message" ("Initial Message")) -> (w189:T14)
        n139 = property class="Pane"(reference=w181, "Origin"=T18 {"Horizontal"=0, "Vertical"=0}) -> ()  [unwired: 1 in, 2 out]
        n140 = control-ref of="This VI"() -> (w179:refnum<vi>)
        n141 = invoke class="VI" method="Default Vals.Reinit All"(reference=w179) -> ()  [unwired: 2 in, 3 out]
        n142 = call-poly "Enqueue Message.vi"("error in (no error)"=w191, "Message"="Init DB", "Message Queue"=w184) -> ("error out"=w192:errorcluster)  [unwired: 7 in, 1 out]
      }
      frame "Init DB" {
        # "open DB"
        # "Install DB file"
        # "create ODBC"
        n143 = call <vilib>:"Application Directory.vi"() -> ("Application Directory"=w200:path)
        n144 = Build Path(base path=w200, name or relative path="data\\config.ini") -> (appended path=w197:path)
        n145 = call <vilib>:"Open Config Data.vi"("configuration file path"=w197) -> ("file created?"=w199:bool, "refnum"=w198:T23)  [unwired: 8 in, 1 out]
        n146 = case shown="True" w199 {
          tunnel: w198 -> [_ w218]
          tunnel: [_ w214] -> w195
          frame False {
          }
          frame True {
            n147 = call "DialogUsingEvents 1.vi"() -> ("Attachment path"=w212:path)  [unwired: 10 in, 1 out]
            n148 = call <vilib>:"Is Path and Not Empty.vi"("path"=w212) -> ("Is Path and Not Empty?"=w213:bool)  [unwired: 4 in]
            n149 = case shown="False" w213 {
              tunnel: [w221 w222] -> w211
              tunnel: w212 -> [_ w222]
              frame False {
                n150 = call <vilib>:"Application Directory.vi"() -> ("Application Directory"=w220:path)
                n151 = Build Path(base path=w220, name or relative path="data\\attachment\\") -> (appended path=w221:path)
              }
              frame True {
              }
            }
            n152 = call-poly <vilib>:"Write Key.vi"("section"="attachment", "value"=w211, "key"="path", "refnum"=w218) -> ("refnum out"=w215:T23)  [unwired: 5 in, 2 out]
            n153 = call <vilib>:"Close Config Data.vi"("refnum"=w215) -> ("error out"=w214:errorcluster)  [unwired: 9 in, 1 out]
          }
        }
        n154 = call-poly <vilib>:"DB Tools Open Connection.vi"("connection information"="Underwriting Pipline Submission") -> ("connection reference"=w207:T24)  [unwired: 7 in, 1 out]
        n155 = call <vilib>:"Open Config Data.vi"("error in (no error)"=w195, "configuration file path"=w197) -> ("refnum"=w196:T23)  [unwired: 7 in, 2 out]
        n156 = call <vilib>:"Application Directory.vi"() -> ("Application Directory"=w204:path)
        n157 = Build Path(base path=w204, name or relative path="data\\attachment\\") -> (appended path=w202:path)
        n158 = call "SQL Commands.vi"("connection reference"=w207) -> ()  [unwired: 9 in, 2 out]
        n159 = call-poly <vilib>:"Read Key.vi"("section"="attachment", "default value"=w202, "key"="path", "refnum"=w196) -> ("value"=w193:path, "refnum out"=w194:T23)  [unwired: 4 in, 2 out]
        n160 = global write "Global.vi" "attachment path"(w193) -> ()
        n161 = call <vilib>:"Close Config Data.vi"("refnum"=w194) -> ()  [unwired: 9 in, 2 out]
      }
      frame "Get login date" {
        # "Something - Replace this message with functionality for your own application."
        n162 = Get Date/Time In Seconds() -> (seconds since 1Jan1904=w229:timestamp)
        n163 = Seconds To Date/Time(time stamp (now)=w229) -> (date time rec=w224:T16)  [unwired: 1 in]
        n164 = Unbundle By Name(w224) -> ("hour"=w228:i32)
        n165 = Greater Or Equal?(x=w228, y=12) -> (x >= y?=w225:bool)
        n166 = case shown="True" w225 {
          tunnel: w224 -> [w234 w238]
          tunnel: [w234 w235] -> w223
          frame False {
          }
          frame True {
            n167 = Unbundle By Name(w238) -> ("day of month"=w237:i32)
            n168 = Increment(x=w237) -> (x+1=w236:i32)
            n169 = Bundle By Name(cluster=w238, "day of month"=w236) -> (w235:T16)
          }
        }
        n170 = Date/Time To Seconds(2:w223) -> (0:w226:timestamp)  [unwired: 1 in]
        n171 = property on="1st Login Date" class="AbsTime (strict)"("Value"=w226) -> ()  [unwired: 2 in, 2 out]
        n172 = Merge Errors(w231) -> (w232:errorcluster)
      }
      frame "Get serial" {
        # "Something - Replace this message with functionality for your own application."
        n173 = Variant To Data(type=Operation_type."Add", Variant=w241) -> (data=w239:T19)  [unwired: 1 in, 1 out]
        n174 = case shown="\"Add\"" w239 {
          tunnel: [w255 w256] -> w244
          frame "Add" {
            n175 = property on="Customer Name" class="Str"() -> ("Value"=w255:string)  [unwired: 2 in, 2 out]
          }
          frame "Query", Default {
            n176 = property on="Customer Name" class="Str"() -> ("Value"=w256:string)  [unwired: 2 in, 2 out]
          }
        }
        n177 = Format Into String(format string="where Customer_Name = '%s'", w244) -> (resulting string=w245:string)  [unwired: 2 in, 1 out]
        n178 = call <userlib>:"DB Interface.vi"("DB Ref In"=w251, "Operation"=DB_Operations_Enum."Select", "condition"=w245, "DB Table"="cases", "DB columns"=string[] ["id"]) -> ("data Out"=w247:variant[][])  [unwired: 7 in, 3 out]
        n179 = call <userlib>:"Variant to String.vi"("Var"=w247) -> ("String"=w242:string)  [unwired: 9 in, 1 out]
        "String" <- w242
        n180 = Merge Errors(w252) -> (w253:errorcluster)
        n181 = case shown="\"Update\"" w239 {
          tunnel: "Case serial : " -> [w260 _ _]
          tunnel: w242 -> [w258 w262 _]
          frame "Add", Default {
            n182 = Concatenate Strings(w260, w258) -> (w259:string)
            n183 = One Button Dialog(message=w259) -> (true=w257:bool)  [unwired: 1 in]
            n184 = case shown="True" w257 {
              frame False {
              }
              frame True {
                n185 = invoke on="Attachement" class="Path" method="Reinit To Default"() -> ()  [unwired: 3 in, 3 out]
                n186 = property on="New Case" class="Clust (strict)"("Value"=T2 {"Customer Number"="", "UW"="", "UWTH"="", "Customer Name"="", "Program"="", "Amount"="", "CCRM"="", "CCRTH"="", "Type"="", "Case status"="Under Review", "1st Login Date"=timestamp(3720200378.523235 s since 1904-01-01), "2nd login Date"=timestamp(0 s since 1904-01-01), "3rd login Date"=timestamp(0 s since 1904-01-01), "Back to business 1"=timestamp(0 s since 1904-01-01), "Back to business 2"=timestamp(0 s since 1904-01-01), "Back to business 3"=timestamp(0 s since 1904-01-01), "Pending risk visit date"=timestamp(0 s since 1904-01-01), "CAM date"=timestamp(0 s since 1904-01-01), "decline date"=timestamp(0 s since 1904-01-01), "CAD submission date"=timestamp(0 s since 1904-01-01), "Comment"="", "Stamped date"=timestamp(0 s since 1904-01-01), "Next Review date"=timestamp(0 s since 1904-01-01), "Declined"="", "Back to business"="", "serial"="", "Business Replay date"=timestamp(0 s since 1904-01-01)} ("New Case")) -> ()  [unwired: 2 in, 2 out]
              }
            }
          }
          frame "Query" {
            n187 = property on="Case Serial 2" class="Str"("Value"=w262) -> ()  [unwired: 2 in, 2 out]
          }
          frame "Update" {
          }
        }
      }
      frame "save new case" {
        n188 = property on="New Case" class="Clust (strict)"() -> ("Value"=w270:T2)  [unwired: 2 in, 2 out]
        n189 = call <userlib>:"Insert to new row in DB.vi"("connection reference"=w268, "Input Cluster"=w270, "table"="cases") -> ("Sucess ?"=w267:bool, "error out"=w264:errorcluster)  [unwired: 5 in, 1 out]
        "error out 2" <- w264
        n190 = Not(x=w264) -> (.not. x?=w266:bool)
        n191 = And(x=w267, y=w266) -> (x .and. y?=w265:bool)
        n192 = case shown="True" w265 {
          tunnel: w264 -> [w277 _]
          tunnel: w263 -> [_ w284]
          frame False {
            w274 = "Duplicate entry"
            n193 = Unbundle By Name(w277) -> ("source"=w276:string)
            n194 = Match Pattern(string=w276, regular expression=w274) -> (match substring=w275:string)  [unwired: 1 in, 3 out]
            n195 = Equal?(x=w275, y=w274) -> (x = y?=w273:bool)
            n196 = case shown="True" w273 {
              frame False {
              }
              frame True {
                n197 = One Button Dialog(message="Customer name must be unique") -> ()  [unwired: 1 in, 1 out]
              }
            }
            n198 = One Button Dialog(message="Error Inserting New Case") -> ()  [unwired: 1 in, 1 out]
          }
          frame True {
            n199 = control-ref of="Customer Name"() -> (w282:refnum<vi>)
            n200 = control-ref of="Attachement"() -> (w286:refnum<vi>)
            n201 = call "Copy attachment to data folder.vi"("Str Refnum"=w282, "Path in"=w286) -> ()  [unwired: 9 in, 1 out]
            n202 = call-poly "Enqueue Message.vi"("Message Data"=Operation_type."Add", "Message"="Get serial", "Message Queue"=w284) -> ("dup Message Queue"=w280:refnum<queue>)  [unwired: 7 in, 1 out]
            n203 = One Button Dialog(message="Case added Successefully") -> ()  [unwired: 1 in, 1 out]
            n204 = call-poly "Enqueue Message.vi"("Message"="Get all Customer names", "Message Queue"=w280) -> ()  [unwired: 8 in, 2 out]
          }
        }
      }
      frame "update case" {
        n205 = property on="Update existing Case" class="Clust (strict)"() -> ("Value"=w290:T9)  [unwired: 2 in, 2 out]
        n206 = property on="Case Serial 2" class="Str"() -> ("Value"=w288:string)  [unwired: 2 in, 2 out]
        n207 = Decimal String To Number(string=w288) -> (number=w289:i32)  [unwired: 2 in, 1 out]
        n208 = call <userlib>:"update data in DB.vi"("connection reference"=w295, "Input Cluster"=w290, "table"="cases", "Unique index"=w289) -> ("Sucess ?"=w294:bool, "error out"=w291:errorcluster)  [unwired: 4 in, 1 out]
        "error out 3" <- w291
        n209 = Not(x=w291) -> (.not. x?=w293:bool)
        n210 = And(x=w294, y=w293) -> (x .and. y?=w292:bool)
        n211 = case shown="True" w292 {
          tunnel: w291 -> [_ _]
          frame False {
            n212 = One Button Dialog(message="Error updating Case") -> ()  [unwired: 1 in, 1 out]
          }
          frame True {
            n213 = disable-structure shown="Enabled" {
              frame Enabled {
                w301 = ""
                n214 = property on="Case Serial 2" class="Str"("Value"=w301) -> ()  [unwired: 2 in, 2 out]
                n215 = property on="attachement" class="Str"("Value"=w301) -> ()  [unwired: 2 in, 2 out]
              }
              frame Disabled {
              }
            }
            n216 = disable-structure shown="Enabled" {
              frame Enabled {
                n217 = invoke on="Update existing Case" class="Clust (strict)" method="Reinit To Default"() -> ()  [unwired: 3 in, 3 out]
              }
              frame Disabled {
              }
            }
            n218 = One Button Dialog(message="Case updated Successefully") -> ()  [unwired: 1 in, 1 out]
          }
        }
      }
      frame "delete case" {
        n219 = property on="Customer Name" class="Str"() -> ("Value"=w302:string)  [unwired: 2 in, 2 out]
        n220 = Format Into String(format string="where Customer_Name ='%s'" ("condition"), w302) -> (resulting string=w303:string)  [unwired: 2 in, 1 out]
        n221 = call <userlib>:"DB Interface.vi"("DB Ref In"=w311, "Operation"=DB_Operations_Enum."Delete", "condition"=w303, "DB Table"="cases") -> ("Sucess ?"=w310:bool, "error out"=w307:errorcluster)  [unwired: 8 in, 2 out]
        "error out 4" <- w307
        n222 = Not(x=w307) -> (.not. x?=w309:bool)
        n223 = And(x=w310, y=w309) -> (x .and. y?=w308:bool)
        n224 = case shown="True" w308 {
          tunnel: w307 -> [_ _]
          frame False {
            n225 = One Button Dialog(message="Error deleting Case") -> ()  [unwired: 1 in, 1 out]
          }
          frame True {
            n226 = disable-structure shown="Enabled" {
              frame Enabled {
                w316 = ""
                n227 = property on="Case Serial 2" class="Str"("Value"=w316) -> ()  [unwired: 2 in, 2 out]
                n228 = property on="attachement" class="Str"("Value"=w316) -> ()  [unwired: 2 in, 2 out]
              }
              frame Disabled {
              }
            }
            n229 = disable-structure shown="Enabled" {
              frame Enabled {
                n230 = invoke on="Update existing Case" class="Clust (strict)" method="Reinit To Default"() -> ()  [unwired: 3 in, 3 out]
              }
              frame Disabled {
              }
            }
            n231 = One Button Dialog(message="Case deleted Successefully") -> ()  [unwired: 1 in, 1 out]
          }
        }
      }
      frame "Query by customer number" {
        n232 = property on="Customer Number" class="Str"() -> ("Value"=w321:string)  [unwired: 2 in, 2 out]
        n233 = control-ref of="Update existing Case"() -> (w318:refnum<vi>)
        n234 = call <userlib>:"Get Data by config name.vi"("config name"=w321, "index"=0, "variant"=w318, "table"="cases", "DB Ref In"=w323) -> ("Array"=w317:string[])  [unwired: 3 in, 3 out]
        n235 = Empty Array?(array=w317) -> (empty?=w320:bool)
        n236 = call "Get dates from DB.vi"("Update existing Case"=w318, "Array"=w317) -> ()  [unwired: 10 in]
        n237 = case shown="False" w320 {
          tunnel: w319 -> [w327 _]
          frame False {
            n238 = call-poly "Enqueue Message.vi"("Message"="Get attachement", "Message Queue"=w327) -> ()  [unwired: 8 in, 2 out]
            n239 = call-poly "Enqueue Message.vi"("Message Data"=Operation_type."Query", "Message"="Get serial", "Message Queue"=w327) -> ()  [unwired: 7 in, 2 out]
          }
          frame True {
            n240 = One Button Dialog(message="Case not found") -> ()  [unwired: 1 in, 1 out]
          }
        }
      }
      frame "Get attachement" {
        n241 = global read "Global.vi" "attachment path"() -> (w333:path)
        n242 = property on="Customer Name" class="Str"() -> ("Value"=w335:string)  [unwired: 2 in, 2 out]
        n243 = call <vilib>:"Is Path and Not Empty.vi"("path"=w333) -> ("Is Path and Not Empty?"=w334:bool)  [unwired: 4 in]
        n244 = case shown="False" w334 {
          tunnel: [w346 w348] -> w332
          tunnel: w333 -> [_ w348]
          frame False {
            n245 = call <vilib>:"Application Directory.vi"() -> ("Application Directory"=w347:path)
            n246 = Build Path(base path=w347, name or relative path="data\\attachment\\") -> (appended path=w346:path)
          }
          frame True {
          }
        }
        n247 = Concatenate Strings(w335, "\\") -> (w340:string)
        n248 = Build Path(base path=w332, name or relative path=w340) -> (appended path=w339:path)
        n249 = List Folder(path=w339) -> (filenames=w338:string[])  [unwired: 3 in, 3 out]
        n250 = Index Array(array=w338, index=0) -> (element=w336:string)
        n251 = property on="attachement" class="Str"("Value"=w336) -> ()  [unwired: 2 in, 2 out]
      }
      frame "Query by customer name" {
        n252 = control-ref of="Update existing Case"() -> (w349:refnum<vi>)
        n253 = property on="Customer Name" class="CmbBox"() -> ("Value"=w353:string)  [unwired: 2 in, 2 out]
        n254 = call <userlib>:"Get Data by config name.vi"("config name"=w353, "index"=3, "variant"=w349, "table"="cases", "DB Ref In"=w355) -> ("Array"=w350:string[])  [unwired: 3 in, 3 out]
        n255 = Empty Array?(array=w350) -> (empty?=w352:bool)
        n256 = call "Get dates from DB.vi"("Update existing Case"=w349, "Array"=w350) -> ()  [unwired: 10 in]
        n257 = case shown="False" w352 {
          tunnel: w351 -> [w359 _]
          frame False {
            n258 = call-poly "Enqueue Message.vi"("Message"="Get attachement", "Message Queue"=w359) -> ()  [unwired: 8 in, 2 out]
            n259 = call-poly "Enqueue Message.vi"("Message Data"=Operation_type."Query", "Message"="Get serial", "Message Queue"=w359) -> ()  [unwired: 7 in, 2 out]
          }
          frame True {
            n260 = One Button Dialog(message="Case not found") -> ()  [unwired: 1 in, 1 out]
          }
        }
      }
      frame "Query by serial" {
        n261 = control-ref of="Update existing Case"() -> (w366:refnum<vi>)
        n262 = property on="Case Serial" class="Str"() -> ("Value"=w365:string)  [unwired: 2 in, 2 out]
        n263 = Decimal String To Number(string=w365) -> (number=w364:i32)  [unwired: 2 in, 1 out]
        n264 = call <userlib>:"Get Config Data.vi"("Unique index"=w364, "variant"=w366, "table"="cases", "DB Ref"=w370) -> ("Array"=w367:string[])  [unwired: 5 in, 2 out]
        n265 = Empty Array?(array=w367) -> (empty?=w369:bool)
        n266 = call "Get dates from DB.vi"("Update existing Case"=w366, "Array"=w367) -> ()  [unwired: 10 in]
        n267 = case shown="True" w369 {
          tunnel: w368 -> [w374 _]
          frame False {
            n268 = call-poly "Enqueue Message.vi"("Message"="Get attachement", "Message Queue"=w374) -> ()  [unwired: 8 in, 2 out]
            n269 = call-poly "Enqueue Message.vi"("Message Data"=Operation_type."Query", "Message"="Get serial", "Message Queue"=w374) -> ()  [unwired: 7 in, 2 out]
          }
          frame True {
            n270 = One Button Dialog(message="Case not found") -> ()  [unwired: 1 in, 1 out]
          }
        }
      }
      frame "Get all Customer names" {
        n271 = call <userlib>:"DB Interface.vi"("DB Ref In"=w391, "Operation"=DB_Operations_Enum."Select", "DB Table"="cases", "DB columns"=string[] ["Customer_Name", "UW"]) -> ("data Out"=w388:variant[][])  [unwired: 8 in, 3 out]
        n272 = Variant To Data(type=string[][] [], Variant=w388) -> (data=w386:string[][])  [unwired: 1 in, 1 out]
        n273 = Index Array(array=w386, index (col) #1=0 ("disabled index (col)"), index (col) #2=1 ("index (col)")) -> (element #1=w384:string[], element #2=w380:string[])  [unwired: 2 in]
        n274 = call-poly <userlib>:"Remove Duplicates from 1D Array__ogtk.vi"("Input Array"=w380) -> ("Output Array"=w379:string[])  [unwired: 1 out]
        n275 = control-ref of="UW"() -> (w382:refnum<vi>)
        n276 = property class="CmbBox"(reference=w382, "Strings[]"=w379) -> (error out=→"error out 10":errorcluster)  [unwired: 1 in, 1 out]
        n277 = property on="Customer Name" class="CmbBox"("Strings[]"=w384) -> ()  [unwired: 2 in, 2 out]
        n278 = property on="UW" class="CmbBox"("Strings[]"=w379) -> ()  [unwired: 2 in, 2 out]
        n279 = property on="UW" class="CmbBox"("Strings[]"=w379) -> ()  [unwired: 2 in, 2 out]
      }
      frame "Generate Report" {
        w396 = "cases" ("DB Table")
        n280 = control-ref of="Report Cluster"() -> (w402:refnum<vi>)
        n281 = disable-structure shown="Enabled" {
          disable-tunnel: w402 -> [w433 _]
          disable-tunnel: [w432 _] -> w401
          frame Enabled {
            n282 = call "get condition.vi"("Report Cluster"=w433) -> ("Condition"=w432:string)  [unwired: 10 in]
          }
          frame Disabled {
          }
        }
        n283 = call <vilib>:"DB Tools List Columns.vi"("table"=w396, "connection reference"=w397) -> ("columns"=w395:string[])  [unwired: 2 in, 3 out]
        "DB Cols Names" <- w395
        n284 = call <userlib>:"DB Interface.vi"("DB Ref In"=w397, "Operation"=DB_Operations_Enum."Select", "condition"=w401, "DB Table"=w396) -> ("data Out"=w403:variant[][], "error out"=→"error out":errorcluster)  [unwired: 8 in, 2 out]
        "data Out" <- w403
        n285 = call <userlib>:"Variant to String 2D Array.vi"("data Out"=w403) -> ("data"=w399:string[][])  [unwired: 9 in, 1 out]
        "data" <- w399
        n286 = Empty Array?(array=w399) -> (empty?=w398:bool)
        n287 = case shown="False" w398 {
          tunnel: w395 -> [w420 _]
          tunnel: w401 -> [w412 _]
          tunnel: w399 -> [w410 _]
          frame False {
            n288 = for {
              tunnel: w410 -> [w422] mode=indexing
              tunnel: [w421] -> w411 mode=indexing
              n289 = for {
                tunnel: w422 -> [w424] mode=indexing
                tunnel: [w423] -> w421 mode=indexing
                n290 = Equal?(x=w424, y="1/1/1904" ("search string")) -> (x = y?=w428:bool)
                n291 = Equal?(x=w424, y="1/1/1600" ("search string")) -> (x = y?=w427:bool)
                n292 = Or(x=w428, y=w427) -> (x .or. y?=w426:bool)
                n293 = Select(t="NULL" ("search string"), s=w426, f=w424) -> (s? t:f=w423:string)
              }
            }
            n294 = call <vilib>:"New Report.vi"("report type"=T21."Excel") -> ("report out"=w408:refnum<class "NI_report.lvclass">)  [unwired: 13 in, 1 out]
            n295 = call <vilib>:"Application Directory.vi"() -> ("Application Directory"=w418:path)
            n296 = Build Path(base path=w418, name or relative path="data\\Reports\\") -> (appended path=w416:path)
            n297 = Concatenate Strings(w412, ".xls") -> (w415:string)
            n298 = Build Path(base path=w416, name or relative path=w415) -> (appended path=w413:path)
            n299 = call-poly <vilib>:"Excel Easy Table.vi"("report in"=w408, "text data"=w411, "column headers"=w420) -> ("report out"=w419:refnum<class "NI_report.lvclass">)  [unwired: 8 in, 4 out]
            n300 = call-dynamic "Save Report to File.vi"("report in"=w419, "report file path"=w413) -> ("error out"=→"error out 6":errorcluster)  [unwired: 12 in, 1 out]
          }
          frame True {
            n301 = One Button Dialog(message="No cases found with these conditions") -> ()  [unwired: 1 in, 1 out]
          }
        }
      }
      frame "Report 2" {
        n302 = call "Get Programs row for daily report.vi"("Refnum in"=w441) -> ("error out"=→"error out 8":errorcluster, "Array out"=w444:string[][])  [unwired: 7 in, 2 out]
        n303 = property on="Case status" class="CmbBox (strict)"() -> ("Strings[]"=w445:string[])  [unwired: 2 in, 2 out]
        n304 = call <vilib>:"New Report.vi"("window state (normal)"=T22."normal", "report type"=T21."Excel") -> ("report out"=w450:refnum<class "NI_report.lvclass">)  [unwired: 12 in, 1 out]
        n305 = Build Array(w445) -> (w453:string[][])
        n306 = call <vilib>:"Application Directory.vi"() -> ("Application Directory"=w461:path)
        n307 = Transpose 2D Array(2D array=w453) -> (transposed array=w452:string[][])
        n308 = Build Path(base path=w461, name or relative path="data\\Reports\\") -> (appended path=w459:path)
        n309 = Index Array(array=w444, index (row)=0) -> (element=w442:string[])  [unwired: 1 in]
        n310 = call-poly <vilib>:"Excel Easy Table.vi"("report in"=w450, "start (0, 0)"=cluster{"row":i32, "column":i32} {"row"=1, "column"=1}, "text data"=w444) -> ("report out"=w446:refnum<class "NI_report.lvclass">, "next cell bottom-left"=w439:cluster{"row":i32, "column":i32})  [unwired: 8 in, 3 out]
        n311 = call-poly <vilib>:"Excel Easy Table.vi"("report in"=w450, "start (0, 0)"=cluster{"row":i32, "column":i32} {"row"=3, "column"=0}, "text data"=w452) -> ("report out"=w462:refnum<class "NI_report.lvclass">)  [unwired: 8 in, 4 out]
        n312 = Concatenate Strings("Daily Report" ("string"), ".xls") -> (w458:string)
        n313 = Build Path(base path=w459, name or relative path=w458) -> (appended path=w456:path)
        n314 = call-dynamic "Save Report to File.vi"("report in"=w462, "report file path"=w456) -> ("error out"=→"error out 7":errorcluster)  [unwired: 12 in, 1 out]
        n315 = for {
          tunnel: w446 -> [w478]
          tunnel: w445 -> [w477] mode=indexing
          tunnel: w442 -> [w469]
          tunnel: w441 -> [w476]
          tunnel: [w475] -> w440 mode=indexing
          shift-right: [w468] -> _
          shift-left: w439 -> [w472]
          tunnel: [w471] -> w438 mode=indexing
          tunnel: [w470] -> w437 mode=indexing
          tunnel: [w467] -> _
          tunnel: "Approved Date" -> [w466]
          tunnel: "decline date" -> [w465]
          n316 = for {
            tunnel: w478 -> [w496]
            tunnel: w469 -> [w492] mode=indexing
            tunnel: w476 -> [w494]
            tunnel: w477 -> [w493]
            shift-right: [w489] -> _
            shift-left: w472 -> [w488]
            tunnel: [w487] -> w475 mode=indexing
            tunnel: [w485] -> w471 mode=indexing
            tunnel: [w484] -> w470 mode=indexing
            tunnel: w469 -> [w483]
            tunnel: [w481] -> w467
            tunnel: w466 -> [w480]
            tunnel: w465 -> [w479]
            i -> [w482]
            n317 = call "even elements.vi"("Numeric"=w482) -> ("Even? (count of program)"=w495:bool)  [unwired: 10 in]
            n318 = case shown="False" w495 {
              tunnel: w488 -> [w506 w538]
              tunnel: w496 -> [w508 w540]
              tunnel: w494 -> [w507 w539]
              tunnel: w493 -> [w500 w528]
              tunnel: w492 -> [w503 _]
              tunnel: [w506 w538] -> w491
              tunnel: [w505 w536] -> w487
              tunnel: [_ w536] -> w485
              tunnel: [_ w527] -> w484
              tunnel: w483 -> [_ w535]
              tunnel: w482 -> [_ w533]
              tunnel: [w504 w532] -> w481
              tunnel: w480 -> [w498 w525]
              tunnel: w479 -> [w497 w526]
              frame True {
                # "Count"
                n319 = case shown="Default" w503 {
                  tunnel: w500 -> [w520 w523]
                  tunnel: [w519 w522] -> w501
                  tunnel: w503 -> [w518 _]
                  frame Default {
                    n320 = Format Into String(format string="SELECT count(id) FROM cases where Case_status = '%s' and Program = '%s'", w520, w518) -> (resulting string=w519:string)  [unwired: 2 in, 1 out]
                  }
                  frame "Grand Total" {
                    n321 = Format Into String(format string="SELECT count(id) FROM cases where Case_status = '%s'", w523) -> (resulting string=w522:string)  [unwired: 2 in, 1 out]
                  }
                }
                n322 = case shown="\"Approved\"" w500 {
                  tunnel: w501 -> [w511 w515 w517]
                  tunnel: [w512 w516 w517] -> w499
                  tunnel: w498 -> [w509 _ _]
                  tunnel: w497 -> [_ w513 _]
                  frame "Approved" {
                    n323 = call "Get condition of date in report.vi"("Date"=w509, "Intial condition"=w511, "Date Label"="CAD submission date") -> ("Condition"=w512:string)  [unwired: 8 in]
                  }
                  frame "Declined" {
                    n324 = call "Get condition of date in report.vi"("Date"=w513, "Intial condition"=w515, "Date Label"="decline date") -> ("Condition"=w516:string)  [unwired: 8 in]
                  }
                  frame Default {
                  }
                }
                n325 = call <userlib>:"DB SQL QRY.vi"("SQL query"=w499, "DB ref in"=w507) -> ("element"=w505:string)  [unwired: 5 in, 4 out]
                n326 = call <vilib>:"Excel Easy Text.vi"("report in"=w508, "border? (F)"=TRUE, "text"=w505, "start (-1, -1)"=w506) -> ("report out"=w504:refnum<class "NI_report.lvclass">)  [unwired: 7 in, 4 out]
              }
              frame False {
                (unwired) 0
                # "Sum"
                n327 = Decrement(x=w533) -> (x-1=w534:i32)
                n328 = Index Array(array=w535, index=w534) -> (element=w531:string)
                n329 = case shown="Default" w531 {
                  tunnel: w528 -> [w552 w555]
                  tunnel: [w551 w554] -> w527
                  tunnel: w531 -> [w550 _]
                  frame Default {
                    n330 = Format Into String(format string="SELECT sum(Amount) FROM cases where Case_status = '%s' and Program = '%s'", w552, w550) -> (resulting string=w551:string)  [unwired: 2 in, 1 out]
                  }
                  frame "Grand Total" {
                    n331 = Format Into String(format string="SELECT sum(Amount) FROM cases where Case_status = '%s'", w555) -> (resulting string=w554:string)  [unwired: 2 in, 1 out]
                  }
                }
                n332 = case shown="\"Approved\"" w528 {
                  tunnel: w527 -> [w543 w547 w549]
                  tunnel: [w544 w548 w549] -> w529
                  tunnel: w526 -> [_ w545 _]
                  tunnel: w525 -> [w541 _ _]
                  frame "Approved" {
                    n333 = call "Get condition of date in report.vi"("Date"=w541, "Intial condition"=w543, "Date Label"="CAD submission date") -> ("Condition"=w544:string)  [unwired: 8 in]
                  }
                  frame "Declined" {
                    n334 = call "Get condition of date in report.vi"("Date"=w545, "Intial condition"=w547, "Date Label"="decline date") -> ("Condition"=w548:string)  [unwired: 8 in]
                  }
                  frame Default {
                  }
                }
                n335 = call <userlib>:"DB SQL QRY.vi"("SQL query"=w529, "DB ref in"=w539) -> ("error out"=→"error out 9":errorcluster, "element"=w536:string)  [unwired: 5 in, 3 out]
                n336 = call <vilib>:"Excel Easy Text.vi"("report in"=w540, "border? (F)"=TRUE, "text"=w536, "start (-1, -1)"=w538) -> ("report out"=w532:refnum<class "NI_report.lvclass">)  [unwired: 7 in, 4 out]
              }
            }
            n337 = Unbundle By Name(w491) -> ("column"=w490:i32)
            n338 = Increment(x=w490) -> (x+1=w486:i32)
            n339 = Bundle By Name(cluster=w491, "column"=w486) -> (w489:cluster{"row":i32, "column":i32})
          }
          n340 = Unbundle By Name(w472) -> ("row"=w473:i32)
          n341 = Increment(x=w473) -> (x+1=w474:i32)
          n342 = Bundle By Name(cluster=w472, "row"=w474) -> (w468:cluster{"row":i32, "column":i32})
        }
        "Array" <- w440
        "Array 2" <- w438
        "Array 3" <- w437
      }
      frame "Generate TAT RISK Report" {
        w564 = "cases" ("DB Table")
        n343 = property on="Program" class="CmbBox (strict)"() -> ("Value"=w557:T3)  [unwired: 2 in, 2 out]
        n344 = Format Into String(format string="where Program = '%s' and Case_status = 'Approved'", w557) -> (resulting string=w558:string)  [unwired: 2 in, 1 out]
        n345 = call <userlib>:"DB Get Columns Names.vi"("Table Name"=w564, "DB ref in"=w565) -> ("DB Cols Names"=w563:string[])  [unwired: 2 in, 7 out]
        "DB Cols Names 2" <- w563
        n346 = call <userlib>:"DB Interface.vi"("DB Ref In"=w565, "Operation"=DB_Operations_Enum."Select", "condition"=w558, "DB Table"=w564) -> ("data Out"=w566:variant[][], "error out"=→"error out 5":errorcluster)  [unwired: 8 in, 2 out]
        "data Out 2" <- w566
        n347 = call <userlib>:"Variant to String 2D Array.vi"("data Out"=w566) -> ("data"=w561:string[][])  [unwired: 9 in, 1 out]
        "data 2" <- w561
        n348 = Empty Array?(array=w561) -> (empty?=w560:bool)
        n349 = case shown="False" w560 {
          tunnel: w563 -> [w585 _]
          tunnel: w561 -> [w576 _]
          frame False {
            n350 = for {
              tunnel: w576 -> [w586] mode=indexing
              tunnel: [w587] -> w577 mode=indexing
              n351 = Index Array(array=w586) -> ()  [unwired: 1 in, 1 out]
              n352 = for {
                tunnel: w586 -> [w589] mode=indexing
                tunnel: [w588] -> w587 mode=indexing
                n353 = Equal?(x=w589, y="1/1/1904" ("search string")) -> (x = y?=w593:bool)
                n354 = Equal?(x=w589, y="1/1/1600" ("search string")) -> (x = y?=w592:bool)
                n355 = Or(x=w593, y=w592) -> (x .or. y?=w591:bool)
                n356 = Select(t="NULL" ("search string"), s=w591, f=w589) -> (s? t:f=w588:string)
              }
            }
            n357 = Get Date/Time In Seconds() -> (seconds since 1Jan1904=w572:timestamp)
            n358 = call <vilib>:"New Report.vi"("report type"=T21."Excel") -> ("report out"=w574:refnum<class "NI_report.lvclass">)  [unwired: 13 in, 1 out]
            n359 = Format Date/Time String(seconds (now)=w572) -> (date/time string=w571:string)  [unwired: 2 in]
            n360 = Concatenate Strings("TAT RISK ", w571) -> (w570:string)
            n361 = call <vilib>:"Application Directory.vi"() -> ("Application Directory"=w583:path)
            n362 = Build Path(base path=w583, name or relative path="data\\Reports\\") -> (appended path=w581:path)
            n363 = Concatenate Strings(w570, ".xls") -> (w580:string)
            n364 = Build Path(base path=w581, name or relative path=w580) -> (appended path=w578:path)
            n365 = call-poly <vilib>:"Excel Easy Table.vi"("report in"=w574, "text data"=w577, "column headers"=w585) -> ("report out"=w584:refnum<class "NI_report.lvclass">)  [unwired: 8 in, 4 out]
            n366 = call-dynamic "Save Report to File.vi"("report in"=w584, "report file path"=w578) -> ()  [unwired: 12 in, 2 out]
          }
          frame True {
            n367 = One Button Dialog(message="No cases found with these conditions") -> ()  [unwired: 1 in, 1 out]
          }
        }
      }
      frame "Something Else" {
        # "Send string to \"Update Display\" message"
        # "#CodeNeeded - Perform whatever actions correspond to the \"Something Else\" message."
        # "Something Else - Replace this message with functionality for your own application."
        n368 = call-poly "Enqueue Message.vi"("error in (no error)"=w602, "Message Data"="\"Do Something Else\" button pressed" ("\"Do Something Else\" button pressed"), "Message"="Update Display", "Message Queue"=w600) -> ("error out"=w601:errorcluster)  [unwired: 6 in, 1 out]
        n369 = Merge Errors(w601) -> (w603:errorcluster)
      }
      frame "Update Display" {
        # "#CodeRecommended - If you wish to decouple the Message Handling Loop from your user interface, consider creating User Events (like the \"Stop\" event in this VI) to message the Event Handling Loop whenever the user interface needs updating."
        # "Update Display - Convert the message data to a string to display in the Data Display indicator."
        n370 = Variant To Data(error in=w610, type="", Variant=w609) -> (data=→"Display <Replace Me>":string, error out=w607:errorcluster)
        n371 = Merge Errors(w607) -> (w611:errorcluster)
      }
      frame "Error" {
        # "#CodeRecommended - If you ever change the name of this \"Error\" message, you'll need to update the name in the Check Loop Error.vi as well."
        # "#CodeRecommended - Consider creating a system for logging errors in some way. These errors are for notification purposes only. Handling of specific errors should be performed in the message frames that generated the error."
        # "Error - Display an error dialog. This message is sent by the \"Error Handler\" VIs at the end of other loops in this application."
        n372 = Variant To Data(error in=w620, type=errorcluster {"status"=FALSE, "code"=0, "source"=""} ("error constant"), Variant=w618) -> (data=w616:errorcluster, error out=w615:errorcluster)
        n373 = call <vilib>:"Simple Error Handler.vi"("error in (no error)"=w616) -> ()  [unwired: 4 in, 5 out]
        n374 = Merge Errors(w615) -> (w614:errorcluster)
      }
      frame "Confirm Quit" {
        # "#CodeNeeded - If you want to provide an \"Are you sure\" dialog (or some other notification) before the application exits, place that code here. This message is typically sent from a Panel Close? event."
        # "Confirm Quit - Message that can confirm whether or not the user wants to exit the application."
        n375 = call-poly "Enqueue Message.vi"("Priority Message? (F)"=TRUE, "error in (no error)"=w628, "Message"="Exit", "Message Queue"=w624) -> ("error out"=w625:errorcluster)  [unwired: 6 in, 1 out]
        n376 = Merge Errors(w625) -> (w626:errorcluster)
      }
      frame "---Copy This Frame---" {
        # "Duplicate this frame when creating new messages.  Change this comment in the duplicated frame to describe this message."
        n377 = Merge Errors(w632) -> (w630:errorcluster)
      }
      frame "Exit" {
        # "Stop the VI"
        # "Release the message queue reference"
        # "#CodeNeeded - Add any required cleanup code here. Note that if 'Exit' was called as a result of an error, an error dialog will be displayed. Add any custom error handling for an 'Exit' condition here as well."
        # "Exit - Exit the application."
        n378 = Variant To Data(type=errorcluster {"status"=FALSE, "code"=0, "source"=""} ("error constant"), Variant=w634) -> (data=w635:errorcluster)  [unwired: 1 in, 1 out]
        n379 = call <vilib>:"Simple Error Handler.vi"("error in (no error)"=w635) -> ()  [unwired: 4 in, 5 out]
        n380 = call "Fire User Event - Stop.vi"("User Event - Stop"=w639) -> ("error out"=w638:errorcluster)  [unwired: 10 in]
        n381 = Release Queue(queue=w644, error in (no error)=w637) -> (error out=w641:errorcluster)  [unwired: 1 in, 2 out]
        n382 = Merge Errors(w638, w641) -> (w640:errorcluster)
      }
      frame Default {
        # "'Default' case only runs if there is a message that isn't defined in any of the other cases.  Output a programming error."
        n383 = xnode "Error Ring"("parameter 0"=w646) -> ("error out"=w647:errorcluster)
      }
    }
    n384 = call "Error Handler - Message Handling Loop.vi"("error in (no error)"=w165, "Message Queue"=w162) -> ("dup error in"=w166:errorcluster)  [unwired: 8 in, 1 out]
  }
  n385 = control-ref of="Update existing Case"() -> ()  [unwired: 1 out]
  n386 = Unregister For Events(event registration refnum=w6, error in=w3) -> (error out=w7:errorcluster)
  n387 = Merge Errors(w7, w11) -> (w8:errorcluster)
  n388 = call "Destroy User Event - Stop.vi"("error in (no error)"=w8, "User Event - Stop"=w1) -> ("error out"=w4:errorcluster)  [unwired: 9 in]
  n389 = disable-structure shown="RUN_TIME_ENGINE==True" {
    disable-tunnel: w4 -> [_ _]
    frame condition #0 (active) {
    }
    frame condition #1 {
      # "Call Quit LabVIEW if running as a built application."
      n390 = Quit LabVIEW() -> ()  [unwired: 1 in]
    }
  }
